vi "main.vi"(0 "Test Pins":T9, 1 "Caller Information":T6, 5 "Test Inputs":T10={"Input Voltage Vin1 in V"=0.0, "Input Voltage Vin2 in V"=0.0, "Duration of the pulse in s"=0.5, "Nominal Output Voltage in V"=0.0, "Ref Voltage level for Settling Time Calc"=0.1, "% of Vnom for Settling Time Calc"=10.0, "Settling Time Calc Option"=enum."Voltage Level ", "Advance Setting"={"Prepare"={"Load SMU Output Function"=enum."VoltageSource"}}, "Save Transient Graph?"=TRUE, "Load Current in A"=0.0, "Save Scope Raw Data?"=FALSE, "Delay - t1 (s)"=0.25, "Delay - t2 (s)"=0.25, "Auto Scale Y-Axis?"=TRUE}, 11 "error in":errorcluster) -> (4 "Test Results":T15 {"Second Edge - Settling Time in s" format="%#.5p"; "First Edge - Settling Time in s" format="%#.5p"; "Actual Sample Rate" format="%#.5g"}, 15 "error out":errorcluster)   [LabVIEW 2020, in "LDO Line Transient.lvlib"]
doc: "<b>Caller</b> Information is input for framework components. Mode should be set to <b>Automation</b> when running from TestStand. Sequence Context should be set to <b>ThisContext</b> when running from TestStand. The values will be updated everytime the setting is applied using \"Edit\" dialog.\n\n<b>Test Pins</b> is names of pins available in the pinmap file. Provide the right pins for the required functionality.\n\n<b>Test Inputs</b> is input required for the measurement to perform.\n\n<b>error in</b> is meant for the sequencing. <b>error in</b> should be <b>no error</b> always.\n\n<b>Test Results</b> contains all the measured data during the measurement and processed results.\n\n<b>error out</b> contains the error occured during measurement.\n\nCheck measurement documentation for more information (<Program Files>\\Soliton Technologies\\MeasurementSuite\\CodeModules\\LDO\\LDO Line Transient.pdf)"
uses:
  LDO Line Transient.lvlib
  Typedefs/Test Results.ctl
  Typedefs/Test Inputs.ctl
  Typedefs/Settling Time Calc Option.ctl
  Typedefs/Advance Settings.ctl
  Typedefs/Adv Settings Setup Instr.ctl
  Reusables/Instrument APIs/Load Output Function.ctl
  <userlib>/_Soliton/Measurement Suite/Reusables/Plugin Common/Typedefs/Caller Events.ctl
  <userlib>/_Soliton/Measurement Suite/Reusables/Plugin Common/Typedefs/Caller Information.ctl
  <userlib>/_Soliton/Measurement Suite/Reusables/Plugin Common/Typedefs/Caller Mode.ctl
  Typedefs/Test Pins.ctl
  Typedefs/Pin Dropdown.ctl
  <userlib>/_Soliton/Measurement Suite/Reusables/Plugin Common/Typedefs/Termination Monitor Info.ctl
  Typedefs/Test Results - Output Voltage Params.ctl
  Typedefs/Test Results - Input Voltage Params.ctl
  Reusables/UI/Progress Monitor/Progress Monitor Option.ctl
  <vilib>/Utility/miscctls.llb/LVMajorAndMinorColorsTypeDef.ctl
  <instrlib>/niDCPower/nidcpower.llb/niDCPower Wait For Event - Event.ctl
  <instrlib>/niDCPower/nidcpower.llb/niDCPower Source Mode.ctl
  <instrlib>/niDCPower/nidcpower.llb/niDCPower Output Function.ctl
  <instrlib>/niScope/Controls/niScope scalar measurement.ctl
  <vilib>/Utility/error.llb/DialogType.ctl
  98935dad-41b4-4920-b943-01b05448cf2f.vi
  d648f1df-a8d9-4085-9eb0-24252e83c66e.vi
  c145c5dd-ae3b-4a85-a29b-a78c16d0dffa.vi
  92dab295-f5c3-455d-a51b-398903a4b680.vi
  64e7d395-4f1e-47d2-aa56-89bf032ac911.vi
  a2cb5138-c738-477a-b5c4-3cdfd9a525fc.vi
  e1ff1980-5b52-43e3-809b-8f211f405b25.vi
  49732470-67c5-4264-8b59-91d7a6bf13ef.vi
  7d547965-4422-4a29-bcba-22e7343550fa.vi
  f054ac9e-285a-43ff-a938-075fc082fc86.vi
  bb3e62c4-a2c2-4505-9438-f842dd651d6c.vi
  ce2ee1e5-697c-4608-b941-8c9b0f21ffd9.vi
  217e438d-a1ad-49ce-9dcd-d015b5ab8206.vi
  20f14550-4756-4008-9ed5-c13eed5fd878.vi
  <userlib>/_Soliton/Measurement Suite/Reusables/InstrumentSessionAPIs/SessionManagerApiPath.vi
  <vilib>/Utility/sysdir.llb/Get System Directory.vi
  <vilib>/Utility/LVLibp/Get Exported File Path.vi
  <userlib>/_Soliton/Measurement Suite/Reusables/Errors/Error 6001.vi
  <instrlib>/niScope/Acquire/Fetch/niScope Multi Fetch Cluster.vi
  <instrlib>/niScope/Measurements/niScope Fetch Measurement.vi
  <userlib>/_Soliton/Measurement Suite/Reusables/Plugin Common/Plugin Common.lvlib
  <userlib>/_Soliton/Measurement Suite/Reusables/Queue Driver/Plugin Queue Driver.lvlib
panel:
  out "Progress":i32(slide) scale=-1.0..0.1
  in  "Terminate":bool
  in  "Run":bool caption="Measure"
  in  "Exit":bool
  out "Header":string
  in  "Tab Enum":T1(radio)
  out "Tab Control":T2(tab)
  in  "SystemSetup":T4={"Set Input Voltage"={"PinStatus"=0, "PinName"="", "Info"=TRUE}, "Measure Input Voltage"={"PinStatus"=0, "PinName"="", "Info"=TRUE}, "Measure Output Voltage"={"PinStatus"=0, "PinName"="", "Info"=TRUE}, "Set Load Current"={"PinStatus"=0, "PinName"="", "Info"=TRUE}}
  out "Sequence Timeout":dbl caption="Sequence Timeout (s)" format="%#.5p"
  in  "Scope Reference Position":dbl format="%#_1f"
  in  "Delay - t2 (s)":dbl=0.25 format="%#_6p"
  in  "Delay - t1 (s)":dbl=0.25 format="%#_6p"
  in  "Load Current (A)":dbl format="%#_6p"
  in  "Voltage to settle above Vnom (V)":dbl=0.1 format="%#_6p"
  in  "Percentage of Vnom (%)":dbl=10.0 caption="Percentage of nominal voltage (%)" format="%#_6f"
  in  "Input Voltage 1 - Vin1 (V)":dbl format="%#_6p"
  in  "Settling Time Calculation":enum32{"Item 0", "Item 1"}(radio)
  in  "Duration of the pulse (s)":dbl=0.5 format="%#_6p"
  in  "Input Voltage 2 - Vin2 (V)":dbl format="%#_6p"
  in  "Nominal Output Voltage (V)":dbl format="%#_6p"
  in  "Advanced Settings":bool
  in  "Auto Scale Y-Axis?":bool=TRUE
  in  "Save Scope Raw Data?":bool=TRUE
  out "Second Edge - Peak Voltage (V)":dbl caption="Peak Voltage (V)" format="%#.6p"
  out "Second Edge - Settling Time (s)":dbl format="%#.5p"
  out "First Edge - Peak Voltage (V)":dbl caption="Peak Voltage (V)" format="%#.6p"
  out "Line Transient":T5(graph)
  in  "Take Transient snapshot?":bool=TRUE
  out "Transient Input Voltage":waveform(dbl)(graph)
  out "Line Transient":T5(graph)
  out "First Edge - Settling Time (s)":dbl format="%#.5p"
  in  "ErrorOccured":errorcluster
  in  "Caller Events":T8
  in  "DataLogPath":path
  # "Supports NIScopeInstrument"
  # "Supports NIScopeInstrument"
  # "Supports NIDCPowerInstrument"
  # "Supports NIDCPowerInstrument"
  # "Settling Time Calculation"
  # "Settling Time is defined as the time taken for the output voltage to recover\nto the LDO nominal output voltage."
  # "Time taken for output voltage to settle to (Choose one below)"
  # "Line Transient"
  # "Output Voltage"
  # "Load SMU"
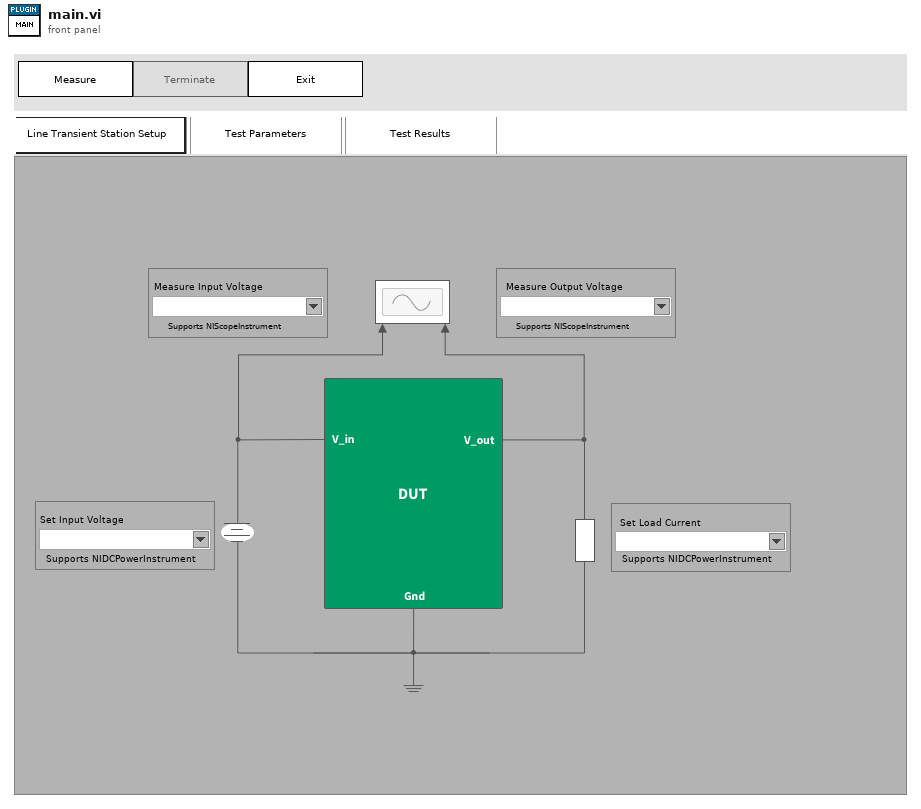
[diagram p1: front panel]
types:
  T1 = enum32{"Station Setup", "Test Parameters", "Test Results"}
  T2 = enum32{"Station Setup", "Test Parameters", "Test Results", "Debug"}
  T3 = typedef "LDO Line Transient.lvlib/Pin Dropdown.ctl" = cluster{"PinStatus":u16, "PinName":string, "Info":bool}
  T4 = cluster{"Set Input Voltage":T3, "Measure Input Voltage":T3, "Measure Output Voltage":T3, "Set Load Current":T3}
  T5 = cluster{"relativeInitialX":dbl, "xIncrement":dbl, "wfm":dbl[]}[]
  T6 = typedef "Plugin Common.lvlib/Caller Information.ctl" = cluster{"Mode":T7, "Sequence Context":refnum<k7>}
  T7 = typedef "Plugin Common.lvlib/Caller Mode.ctl" = enum16{"Standalone", "Automation", "MeasurementSuite"}
  T8 = typedef "Plugin Common.lvlib/Caller Events.ctl" = cluster{"Caller Event":refnum<user-event>}
  T9 = typedef "LDO Line Transient.lvlib/Test Pins.ctl" = cluster{"Set Input Voltage":string, "Set Load Current":string, "Measure Input Voltage":string, "Measure Output Voltage":string}
  T10 = typedef "LDO Line Transient.lvlib/Test Inputs.ctl" = cluster{"Input Voltage Vin1 in V":dbl, "Input Voltage Vin2 in V":dbl, "Duration of the pulse in s":dbl, "Nominal Output Voltage in V":dbl, "Ref Voltage level for Settling Time Calc":dbl, "% of Vnom for Settling Time Calc":dbl, "Settling Time Calc Option":T11, "Advance Setting":T12, "Save Transient Graph?":bool, "Load Current in A":dbl, "Save Scope Raw Data?":bool, "Delay - t1 (s)":dbl, "Delay - t2 (s)":dbl, "Auto Scale Y-Axis?":bool}
  T11 = typedef "LDO Line Transient.lvlib/Settling Time Calc Option.ctl" = enum16{"Voltage Level ", "Percentage of Vnom"}
  T12 = typedef "LDO Line Transient.lvlib/Advance Settings.ctl" = cluster{"Prepare":T13}
  T13 = typedef "LDO Line Transient.lvlib/Adv Settings Setup Instr.ctl" = cluster{"Load SMU Output Function":T14}
  T14 = typedef "Load Output Function.ctl" = enum16{"VoltageSource", "CurrentSource"}
  T15 = typedef "LDO Line Transient.lvlib/Test Results.ctl" = cluster{"Output Voltage Measured":cluster{"relativeInitialX":dbl, "xIncrement":dbl, "wfm":dbl[]}, "Input Voltage Measured":cluster{"relativeInitialX":dbl, "xIncrement":dbl, "wfm":dbl[]}, "Actual Sample Rate":dbl, "First Edge - Settling Time in s":dbl, "Second Edge - Settling Time in s":dbl}
  T16 = typedef "Plugin Common.lvlib/Termination Monitor Info.ctl" = cluster{"Caller Information":T6, "Execution":refnum<k7>, "Termination Monitor":refnum<k7>, "Type":string, "Plugin Name":string}
  T17 = typedef "LDO Line Transient.lvlib/Test Results - Output Voltage Params.ctl" = cluster{"First Edge - Settling Time (s)":dbl, "First Edge - Peak Voltage (V)":dbl, "Second Edge - Settling Time (s)":dbl, "Second Edge - Peak Voltage (V)":dbl, "Vmax":dbl, "Vmin":dbl}
  T18 = typedef "LDO Line Transient.lvlib/Test Results - Input Voltage Params.ctl" = cluster{"Vmax":dbl, "Vmin":dbl}
  T19 = cluster{"Termination Monitor Info":T16, "Test Inputs":T10, "Test Results":T15, "Test Results[][]":string[][], "Test Pins":T9, "Logger Folder Path":path, "Valid Logger Path?":bool, "Logger File Path":path, "Waveform for settling time analysis":dbl[], "Min delay for Reference Position":u32, "Output Voltage Coupling":i32, "Input Voltage Waveform":dbl[], "Input Voltage Source Delay":dbl[], "Output Voltage Params":T17, "Input Voltage Params":T18, "UI Ctls":refnum<vi>[]}
  T20 = typedef "Progress Monitor Option.ctl" = enum16{"State Array Init", "Get State Index"}
  T21 = enum8{"Enabled", "Disabled", "Disabled and Grayed Out"}
  T22 = cluster{"Set Iload":T3, "Set Vin":T3, "Capture Vout":T3, "Capture Vin":T3}
  T23 = typedef "LVMajorAndMinorColorsTypeDef.ctl" = cluster{"Major Color":u32, "Minor Color":u32}
  T24 = cluster{"relativeInitialX":dbl, "xIncrement":dbl, "wfm":dbl[]}
  T25 = typedef "niDCPower Wait For Event - Event.ctl" = i32
  T26 = typedef "niDCPower Output Function.ctl" = i32
  T27 = typedef "niDCPower Source Mode.ctl" = i32
  T28 = typedef "niScope scalar measurement.ctl" = i32
  T29 = typedef "DialogType.ctl" = u16
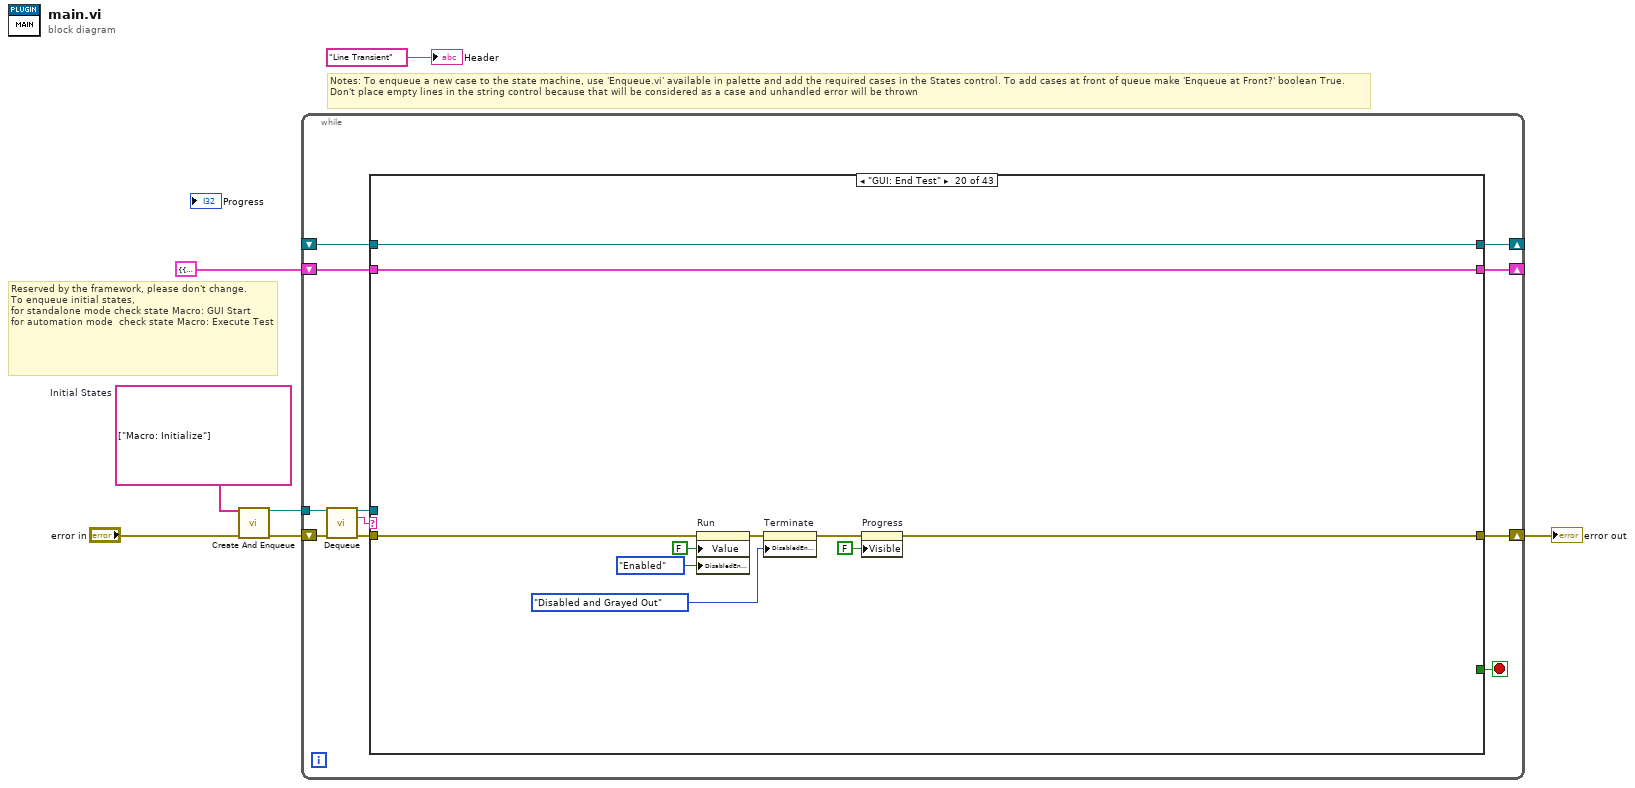
[diagram p0: block diagram]
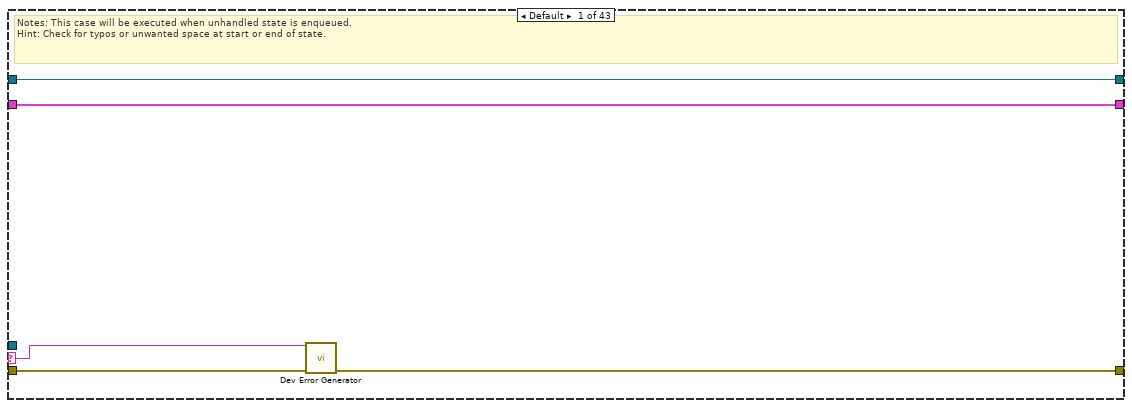
[diagram p2: hidden frame]
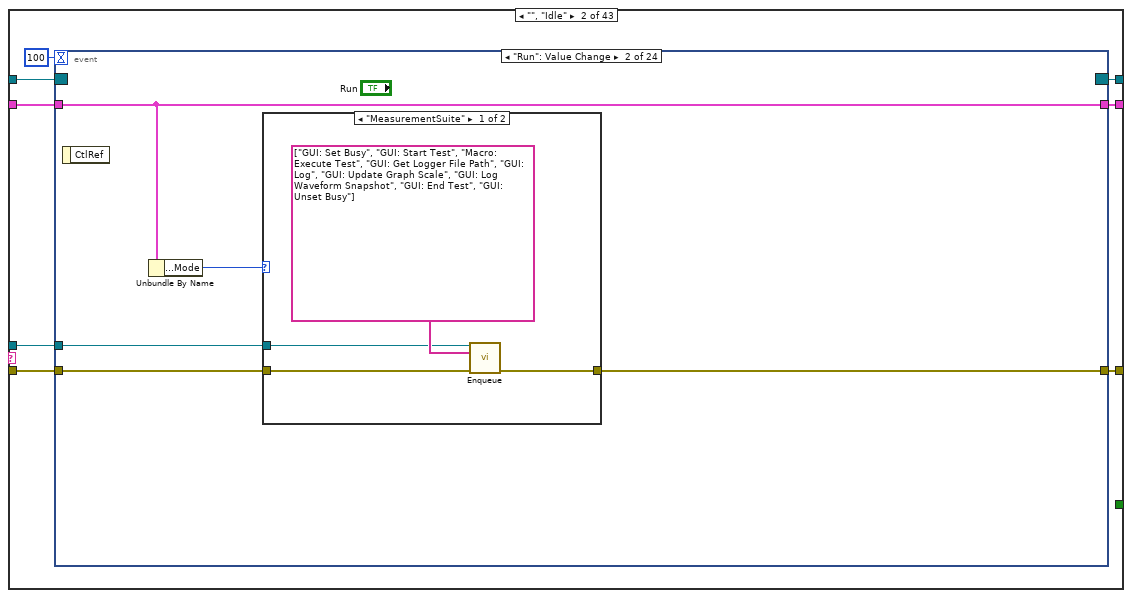
[diagram p3: hidden frame]
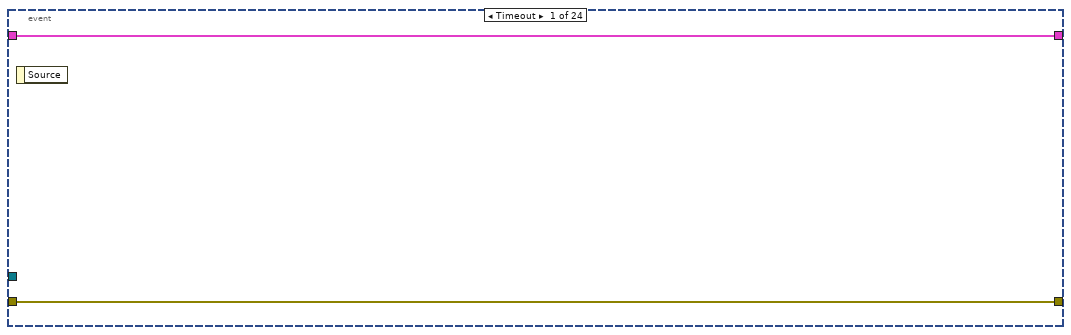
[diagram p4: hidden frame]
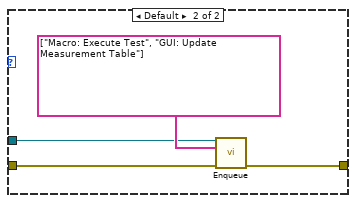
[diagram p5: hidden frame]
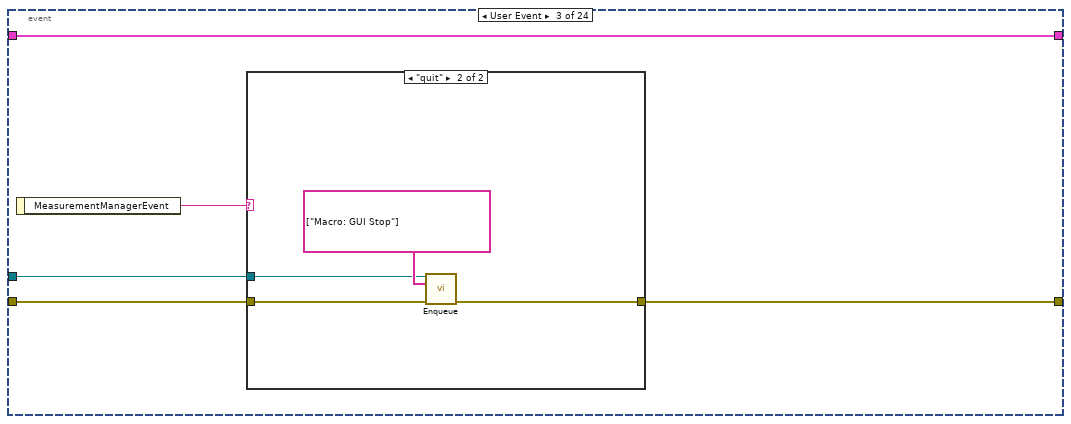
[diagram p6: hidden frame]
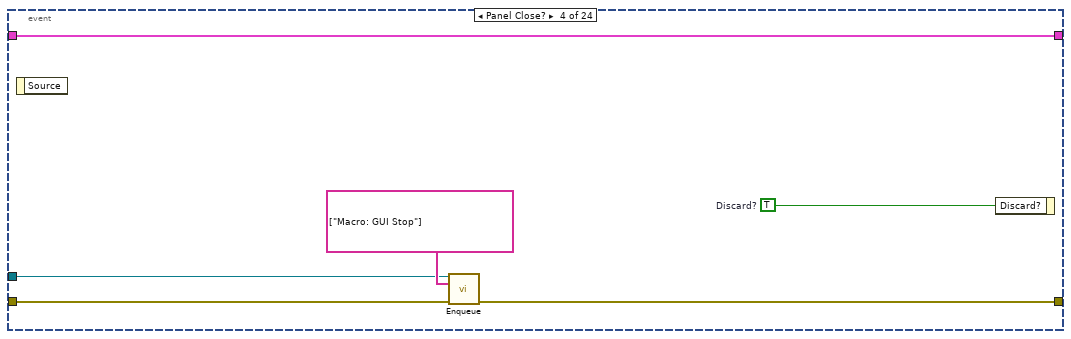
[diagram p8: hidden frame]
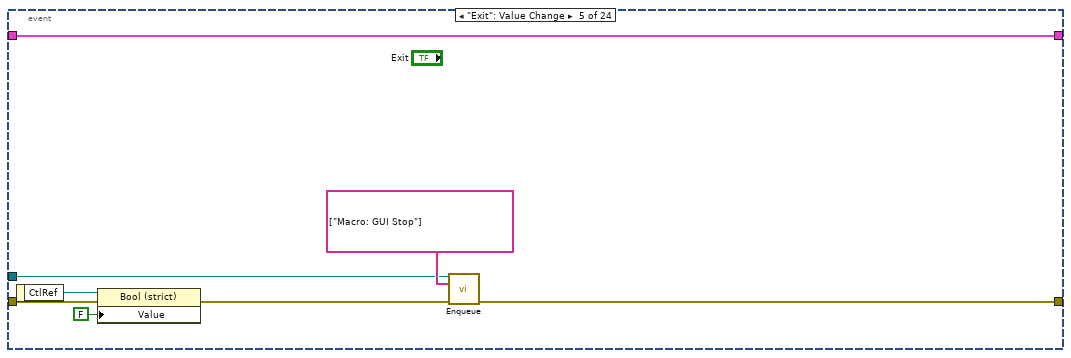
[diagram p9: hidden frame]
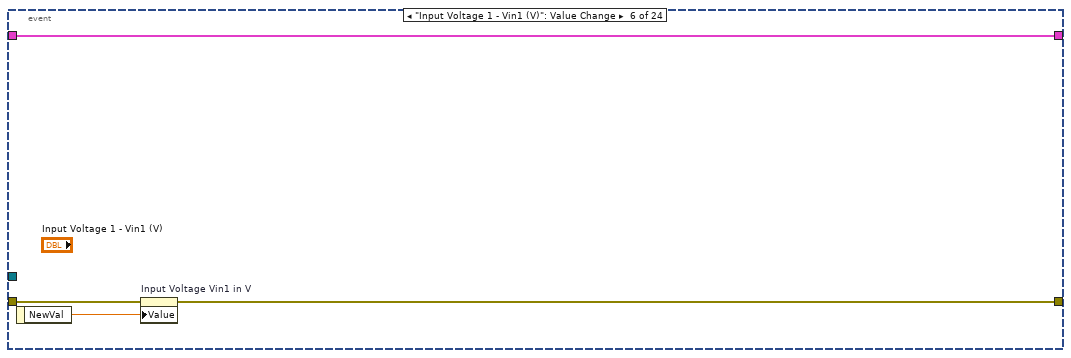
[diagram p10: hidden frame]
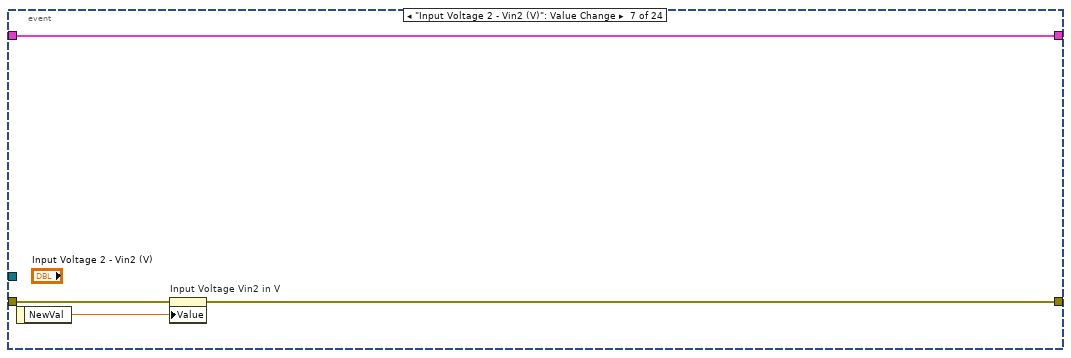
[diagram p11: hidden frame]
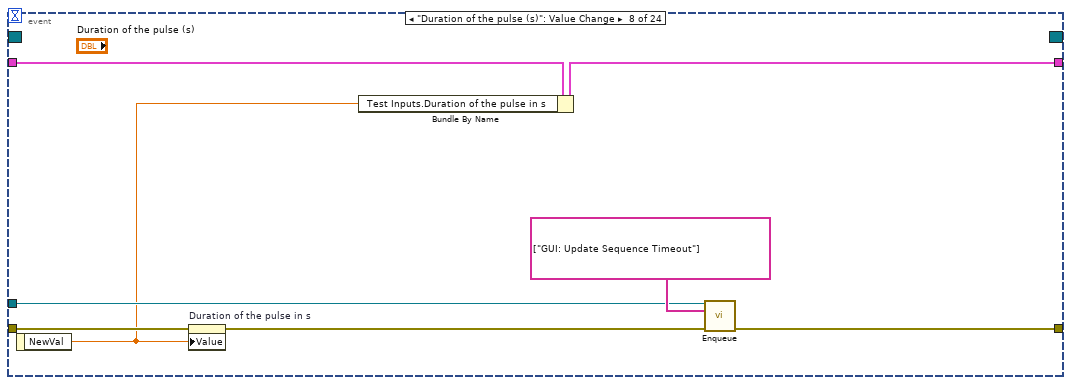
[diagram p12: hidden frame]
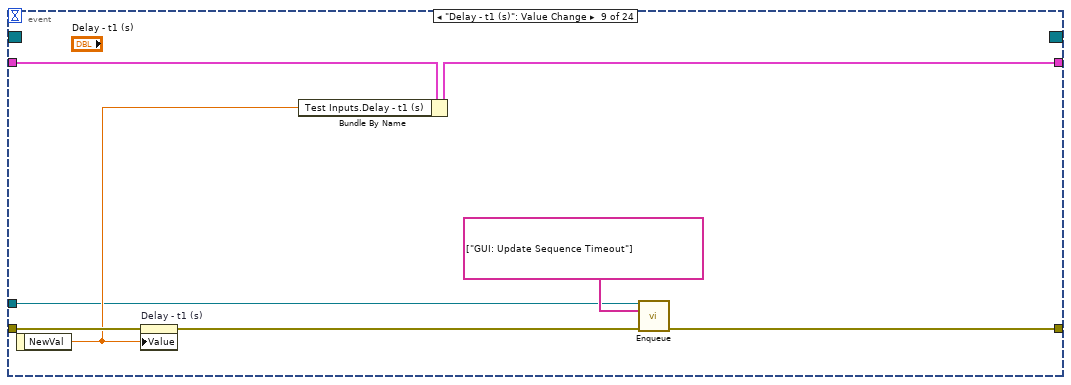
[diagram p13: hidden frame]
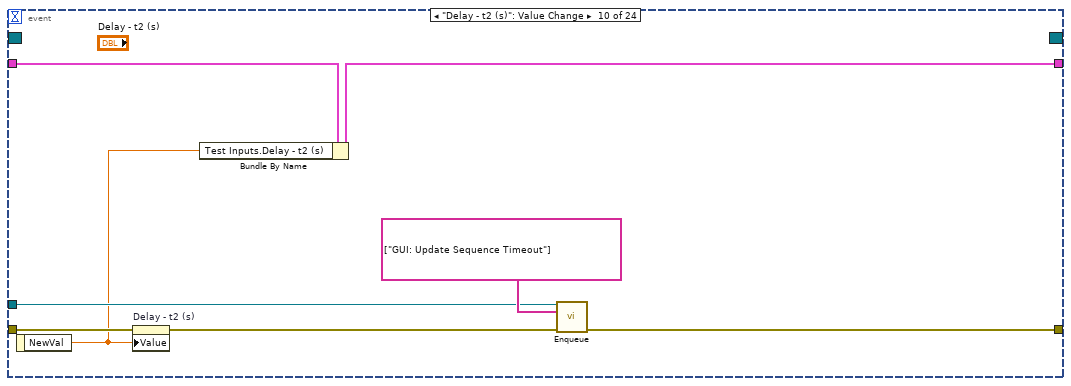
[diagram p14: hidden frame]
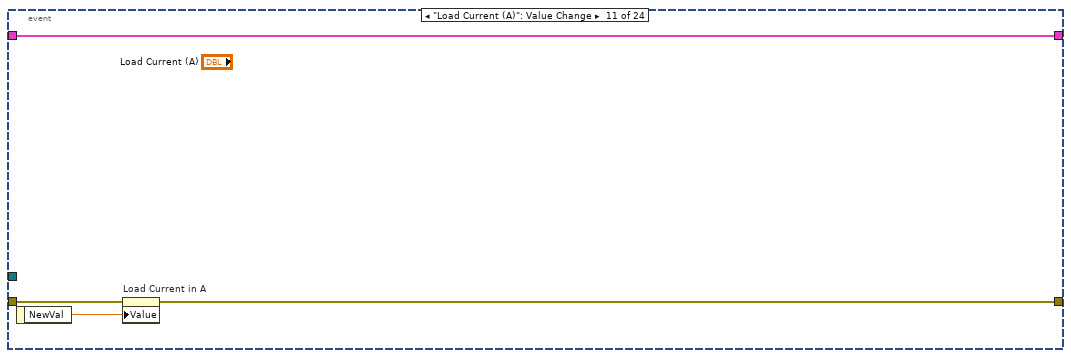
[diagram p15: hidden frame]
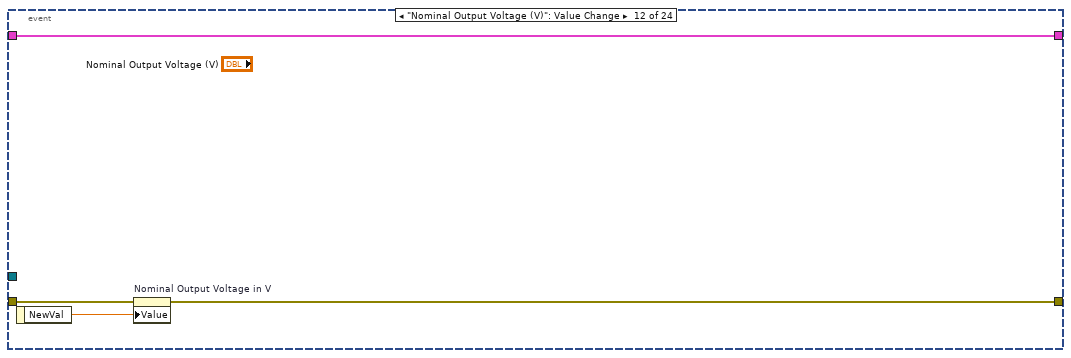
[diagram p16: hidden frame]
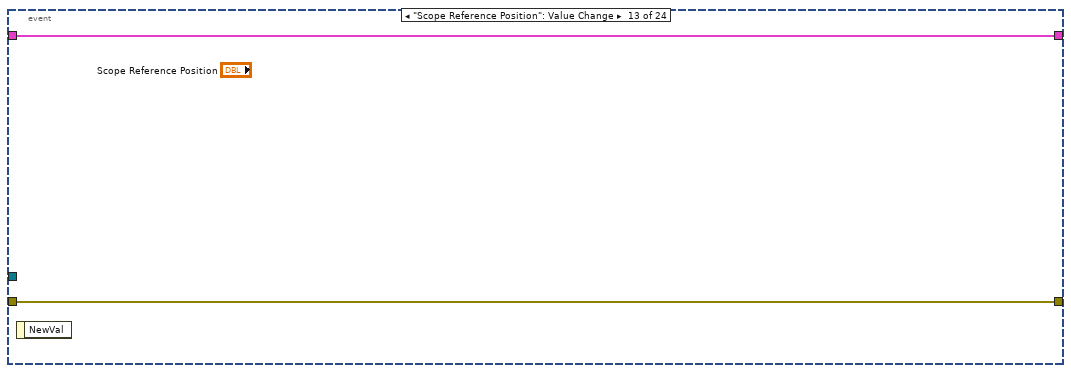
[diagram p17: hidden frame]
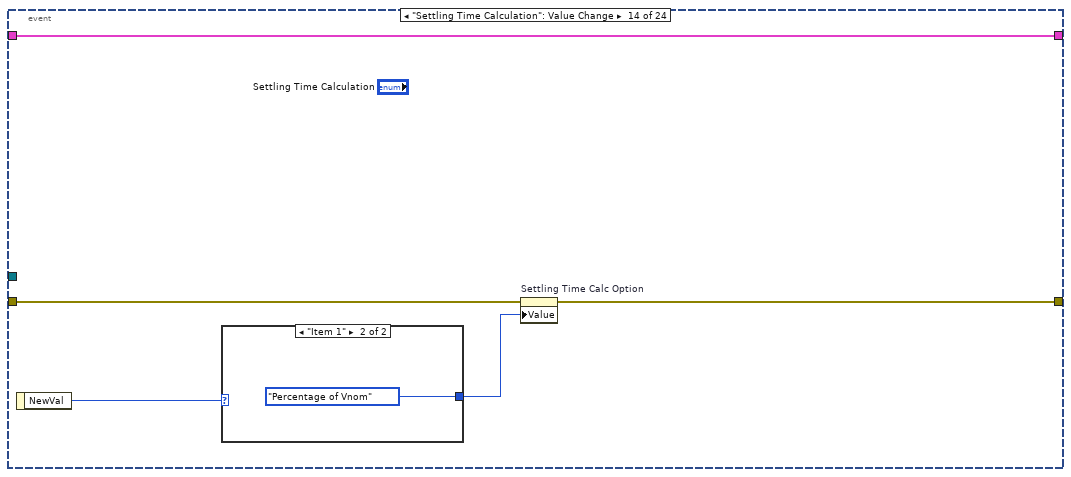
[diagram p18: hidden frame]
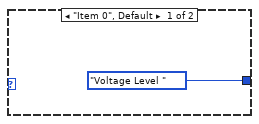
[diagram p19: hidden frame]
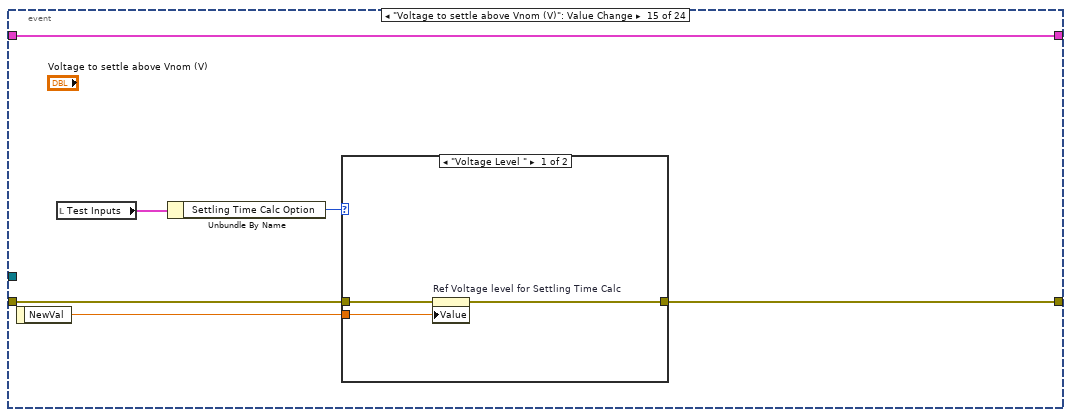
[diagram p20: hidden frame]
diagram:
  w7 = string[] ["Macro: Initialize"]  # Initial States
  # "Notes: To enqueue a new case to the state machine, use 'Enqueue.vi' available in palette and add the required cases in the States control. To add cases at front of queue make 'Enqueue at Front?' boolean True. Don't place empty lines in the string control because that will be considered as a case and unhandled error will be thrown"
  # "Reserved by the framework, please don't change. \nTo enqueue initial states,\nfor standalone mode check state Macro: GUI Start\nfor automation mode  check state Macro: Execute Test"
  n1 = call <userlib>:"Create And Enqueue.vi"("Initial States"=w7, "error in (no error)"="error in") -> ("Queue out"=w5:refnum<queue>, "error out"=w3:errorcluster)  [unwired: 12 in]
  n2 = while {
    shift-right: [w18] -> w4
    shift-left: w3 -> [w16]
    shift-right: [w14] -> _
    shift-left: T19 {"Termination Monitor Info"={"Caller Information"={"Mode"=enum."Standalone", "Sequence Context"=refnum}, "Execution"=refnum, "Termination Monitor"=refnum, "Type"="", "Plugin Name"=""}, "Test Inputs"={"Input Voltage Vin1 in V"=0.0, "Input Voltage Vin2 in V"=0.0, "Duration of the pulse in s"=0.0, "Nominal Output Voltage in V"=0.0, "Ref Voltage level for Settling Time Calc"=0.0, "% of Vnom for Settling Time Calc"=0.0, "Settling Time Calc Option"=enum."Voltage Level ", "Advance Setting"={"Prepare"={"Load SMU Output Function"=enum."VoltageSource"}}, "Save Transient Graph?"=FALSE, "Load Current in A"=0.0, "Save Scope Raw Data?"=FALSE, "Delay - t1 (s)"=0.0, "Delay - t2 (s)"=0.0, "Auto Scale Y-Axis?"=FALSE}, "Test Results"={"Output Voltage Measured"={"relativeInitialX"=0.0, "xIncrement"=0.0, "wfm"=[]}, "Input Voltage Measured"={"relativeInitialX"=0.0, "xIncrement"=0.0, "wfm"=[]}, "Actual Sample Rate"=0.0, "First Edge - Settling Time in s"=0.0, "Second Edge - Settling Time in s"=0.0}, "Test Results[][]"=[], "Test Pins"={"Set Input Voltage"="", "Set Load Current"="", "Measure Input Voltage"="", "Measure Output Voltage"=""}, "Logger Folder Path"=path "", "Valid Logger Path?"=FALSE, "Logger File Path"=path "", "Waveform for settling time analysis"=[], "Min delay for Reference Position"=0, "Output Voltage Coupling"=0, "Input Voltage Waveform"=[], "Input Voltage Source Delay"=[], "Output Voltage Params"={"First Edge - Settling Time (s)"=0.0, "First Edge - Peak Voltage (V)"=0.0, "Second Edge - Settling Time (s)"=0.0, "Second Edge - Peak Voltage (V)"=0.0, "Vmax"=0.0, "Vmin"=0.0}, "Input Voltage Params"={"Vmax"=0.0, "Vmin"=0.0}, "UI Ctls"=[]} -> [w13]
    tunnel: w5 -> [w12]
    shift-right: [w9] -> _
    shift-left: _ -> [w10]
    stop <- w17 stop-if-true
    n3 = call <userlib>:"Dequeue.vi"("Queue in"=w12, "error in (no error)"=w16) -> ("Queue out"=w11:refnum<queue>, "Dequeued State"=w8:string, "error out"=w15:errorcluster)  [unwired: 11 in]
    n4 = case shown="\"GUI: End Test\"" w8 {
      selector: w8 -> [w21 _ _ _ _ _ _ _ _ _ _ _ _ _ _ _ w423 w439 _ _ _ _ _ _ _ w508 w529 w541 w574 w588 w598 w615 w673 w701 w732 w756 w777 w806 w825 w830 _ _ _]
      tunnel: w15 -> [w20 w28 w227 w236 w251 w257 w264 w269 w312 w323 w327 w330 w334 w363 w378 w389 w424 w440 w456 w467 w476 w487 w492 w499 w504 w506 w530 w542 w575 w589 w599 w616 w674 w702 w733 w757 w778 w807 w826 w831 w838 w845 w863]
      tunnel: [w22 w29 w227 w239 w247 w258 w265 w269 w292 w321 w325 w330 w333 w364 w376 w390 w428 w444 w457 w468 w475 w487 w493 w500 w504 w509 w533 w540 w563 w590 w607 w634 w689 w721 w734 w758 w772 w795 w824 w832 w838 w843 w857] -> w18
      tunnel: [_ _ _ _ _ _ _ _ _ _ _ _ _ _ _ _ _ _ _ _ _ _ _ _ _ _ _ _ _ _ _ _ _ _ _ _ _ _ _ _ _ w840 TRUE] -> w17
      tunnel: [w23 w31 w226 w229 w252 w259 w266 w268 w289 w322 w326 w329 w332 w365 w382 w388 w427 w443 w464 w474 w477 w486 w491 w498 w503 w512 w535 w545 w556 w593 w606 w624 w687 w718 w737 w761 w792 w811 w828 w835 w837 w842 w864] -> w14
      tunnel: w13 -> [w23 w30 w226 w240 w252 w259 w266 w268 w317 w322 w326 w329 w331 w365 w382 w388 w427 w443 w464 w474 w477 w486 w490 w497 w503 w519 w535 w545 w555 w592 w606 w623 w686 w717 w736 w760 w792 w811 w828 w835 w837 w842 w864]
      tunnel: w11 -> [_ w24 _ w238 w250 w255 w262 _ _ _ _ _ _ _ _ _ _ _ _ _ _ _ _ _ _ _ _ _ _ _ _ _ _ _ _ _ _ _ _ _ _ w839 w862]
      tunnel: w10 -> [w19 w26 w225 w237 w249 w254 w261 w267 w316 _ w324 w328 w339 w366 w383 w395 w434 w450 w463 w473 w484 w485 w494 w501 w502 w517 w536 w546 w583 w597 w614 w638 w698 w731 w743 w762 w793 w817 w829 w834 w836 w844 w861]
      tunnel: [w19 w25 w225 w237 w249 w254 w261 w267 w316 w320 w324 w328 w339 w366 w383 w395 w434 w450 w463 w473 w484 w485 w494 w501 w502 w517 w536 w546 w583 w597 w614 w638 w698 w731 w743 w762 w793 w817 w829 w834 w836 w844 w861] -> w9
      frame Default {
        # "Notes: This case will be executed when unhandled state is enqueued. \nHint: Check for typos or unwanted space at start or end of state."
        n5 = call <userlib>:"Dev Error Generator.vi"("State"=w21, "error in (no error)"=w20) -> ("error out"=w22:errorcluster)  [unwired: 13 in]
      }
      frame "", "Idle" {
        n6 = event shown="[1] \"Run\": Value Change" {
          selector: w26 -> [_ _ _ _ _ _ _ _ _ _ _ _ _ _ _ _ _ _ _ _ _ _ _ _]
          dyn-events: [_ _ _ _ _ _ _ _ _ _ _ _ _ _ _ _ _ _ _ _ _ _ _ _] -> w25
          timeout: 100 -> [_ _ _ _ _ _ _ _ _ _ _ _ _ _ _ _ _ _ _ _ _ _ _ _]
          tunnel: [w33 w35 w51 w62 w70 w74 w78 w81 w93 w96 w106 w110 w112 w117 w125 w136 w147 w151 w155 w158 w174 w212 w217 w222] -> w31
          tunnel: w30 -> [w33 w35 w51 w62 w70 w74 w78 w80 w92 w95 w106 w110 w112 w117 w125 w136 w147 w151 w155 w162 w173 w211 w217 w221]
          tunnel: [w32 w38 w49 w59 w68 w73 w77 w83 w88 w99 w104 w109 w111 w114 w123 w133 w145 w149 w153 w160 w176 w191 w216 w219] -> w29
          tunnel: w28 -> [w32 w37 w50 w58 w67 w72 w76 w86 w94 w102 w105 w108 w111 w115 w124 w132 w146 w150 w154 w159 w177 w187 w216 w224]
          tunnel: w24 -> [_ w36 w47 w57 w66 _ _ w82 w87 w98 _ _ _ _ _ _ _ _ _ _ _ _ _ _]
          event Timeout {
            n7 = event-data() -> ()  [unwired: 1 in, 1 out]
          }
          event "Run": Value Change {
            n8 = event-data() -> ()  [unwired: 1 in, 1 out]
            n9 = Unbundle By Name(w35) -> ("Termination Monitor Info.Caller Information.Mode"=w34:T7)
            n10 = case shown="\"MeasurementSuite\"" w34 {
              tunnel: [w41 w45] -> w38
              tunnel: w37 -> [w40 w44]
              tunnel: w36 -> [w39 w43]
              frame "MeasurementSuite" {
                n11 = call <userlib>:"Enqueue.vi"("Queue in"=w39, "States"=string[] ["GUI: Set Busy", "GUI: Start Test", "Macro: Execute Test", "GUI: Get Logger File Path", "GUI: Log", "GUI: Update Graph Scale", "GUI: Log Waveform Snapshot", "GUI: End Test", "GUI: Unset Busy"], "error in (no error)"=w40) -> ("error out"=w41:errorcluster)  [unwired: 11 in, 1 out]
              }
              frame Default {
                n12 = call <userlib>:"Enqueue.vi"("Queue in"=w43, "States"=string[] ["Macro: Execute Test", "GUI: Update Measurement Table"], "error in (no error)"=w44) -> ("error out"=w45:errorcluster)  [unwired: 11 in, 1 out]
              }
            }
          }
          event User Event {
            n13 = event-data() -> ("MeasurementManagerEvent"=w48:string)  [unwired: 1 in]
            n14 = case shown="\"quit\"" w48 {
              tunnel: [w52 w53] -> w49
              tunnel: w50 -> [w52 w55]
              tunnel: w47 -> [_ w54]
              frame Default {
              }
              frame "quit" {
                n15 = call <userlib>:"Enqueue.vi"("Queue in"=w54, "States"=string[] ["Macro: GUI Stop"], "error in (no error)"=w55) -> ("error out"=w53:errorcluster)  [unwired: 11 in, 1 out]
              }
            }
          }
          event Panel Close? {
            w61 = TRUE  # Discard?
            n16 = event-data() -> ()  [unwired: 1 in, 1 out]
            n17 = call <userlib>:"Enqueue.vi"("Queue in"=w57, "States"=string[] ["Macro: GUI Stop"], "error in (no error)"=w58) -> ("error out"=w59:errorcluster)  [unwired: 11 in, 1 out]
            n18 = event-data("Discard?"=w61) -> ()  [unwired: 1 in, 1 out]
          }
          event "Exit": Value Change {
            n19 = event-data() -> ("CtlRef"=w64:refnum<vi>)  [unwired: 1 in]
            n20 = property class="Bool (strict)"(reference=w64, error in=w67, "Value"=FALSE) -> (error out=w65:errorcluster)  [unwired: 1 out]
            n21 = call <userlib>:"Enqueue.vi"("Queue in"=w66, "States"=string[] ["Macro: GUI Stop"], "error in (no error)"=w65) -> ("error out"=w68:errorcluster)  [unwired: 11 in, 1 out]
          }
          event "Input Voltage 1 - Vin1 (V)": Value Change {
            n22 = event-data() -> ("NewVal"=w71:dbl)  [unwired: 1 in]
            n23 = property on="Input Voltage Vin1 in V" class="DigNum (strict)"(error in=w72, "Value"=w71) -> (error out=w73:errorcluster)  [unwired: 1 in, 1 out]
          }
          event "Input Voltage 2 - Vin2 (V)": Value Change {
            n24 = event-data() -> ("NewVal"=w75:dbl)  [unwired: 1 in]
            n25 = property on="Input Voltage Vin2 in V" class="DigNum (strict)"(error in=w76, "Value"=w75) -> (error out=w77:errorcluster)  [unwired: 1 in, 1 out]
          }
          event "Duration of the pulse (s)": Value Change {
            n26 = event-data() -> ("NewVal"=w79:dbl)  [unwired: 1 in]
            n27 = property on="Duration of the pulse in s" class="DigNum (strict)"(error in=w86, "Value"=w79) -> (error out=w84:errorcluster)  [unwired: 1 in, 1 out]
            n28 = Bundle By Name(cluster=w80, "Test Inputs.Duration of the pulse in s"=w79) -> (w81:T19)
            n29 = call <userlib>:"Enqueue.vi"("Queue in"=w82, "States"=string[] ["GUI: Update Sequence Timeout"], "error in (no error)"=w84) -> ("error out"=w83:errorcluster)  [unwired: 11 in, 1 out]
          }
          event "Delay - t1 (s)": Value Change {
            n30 = event-data() -> ("NewVal"=w91:dbl)  [unwired: 1 in]
            n31 = property on="Delay - t1 (s)" class="DigNum (strict)"(error in=w94, "Value"=w91) -> (error out=w89:errorcluster)  [unwired: 1 in, 1 out]
            n32 = Bundle By Name(cluster=w92, "Test Inputs.Delay - t1 (s)"=w91) -> (w93:T19)
            n33 = call <userlib>:"Enqueue.vi"("Queue in"=w87, "States"=string[] ["GUI: Update Sequence Timeout"], "error in (no error)"=w89) -> ("error out"=w88:errorcluster)  [unwired: 11 in, 1 out]
          }
          event "Delay - t2 (s)": Value Change {
            n34 = event-data() -> ("NewVal"=w97:dbl)  [unwired: 1 in]
            n35 = property on="Delay - t2 (s)" class="DigNum (strict)"(error in=w102, "Value"=w97) -> (error out=w100:errorcluster)  [unwired: 1 in, 1 out]
            n36 = Bundle By Name(cluster=w95, "Test Inputs.Delay - t2 (s)"=w97) -> (w96:T19)
            n37 = call <userlib>:"Enqueue.vi"("Queue in"=w98, "States"=string[] ["GUI: Update Sequence Timeout"], "error in (no error)"=w100) -> ("error out"=w99:errorcluster)  [unwired: 11 in, 1 out]
          }
          event "Load Current (A)": Value Change {
            n38 = event-data() -> ("NewVal"=w103:dbl)  [unwired: 1 in]
            n39 = property on="Load Current in A" class="DigNum (strict)"(error in=w105, "Value"=w103) -> (error out=w104:errorcluster)  [unwired: 1 in, 1 out]
          }
          event "Nominal Output Voltage (V)": Value Change {
            n40 = event-data() -> ("NewVal"=w107:dbl)  [unwired: 1 in]
            n41 = property on="Nominal Output Voltage in V" class="DigNum (strict)"(error in=w108, "Value"=w107) -> (error out=w109:errorcluster)  [unwired: 1 in, 1 out]
          }
          event "Scope Reference Position": Value Change {
            n42 = event-data() -> ()  [unwired: 1 in, 1 out]
          }
          event "Settling Time Calculation": Value Change {
            n43 = event-data() -> ("NewVal"=w116:enum32{"Item 0", "Item 1"})  [unwired: 1 in]
            n44 = case shown="\"Item 1\"" w116 {
              tunnel: [Settling_Time_Calc_Option."Voltage Level " ("Value") Settling_Time_Calc_Option."Percentage of Vnom" ("Value")] -> w113
              frame "Item 0", Default {
              }
              frame "Item 1" {
              }
            }
            n45 = property on="Settling Time Calc Option" class="Enum (strict)"(error in=w115, "Value"=w113) -> (error out=w114:errorcluster)  [unwired: 1 in, 1 out]
          }
          event "Voltage to settle above Vnom (V)": Value Change {
            n46 = event-data() -> ("NewVal"=w120:dbl)  [unwired: 1 in]
            n47 = local read "Test Inputs"() -> (w122:T10)
            n48 = Unbundle By Name(w122) -> ("Settling Time Calc Option"=w121:T11)
            n49 = case shown="\"Voltage Level \"" w121 {
              tunnel: w124 -> [w128 w129]
              tunnel: [w127 w129] -> w123
              tunnel: w120 -> [w126 _]
              frame "Voltage Level " {
                n50 = property on="Ref Voltage level for Settling Time Calc" class="DigNum (strict)"(error in=w128, "Value"=w126) -> (error out=w127:errorcluster)  [unwired: 1 in, 1 out]
              }
              frame "Percentage of Vnom", Default {
              }
            }
          }
          event "Percentage of Vnom (%)": Value Change {
            # "#TODO\nDo this logic when executing the testw"
            n51 = event-data() -> ("NewVal"=w131:dbl)  [unwired: 1 in]
            n52 = local read "Test Inputs"() -> (w134:T10)
            n53 = Unbundle By Name(w134) -> ("Settling Time Calc Option"=w135:T11, "Nominal Output Voltage in V"=w130:dbl)
            n54 = case shown="\"Percentage of Vnom\"" w135 {
              tunnel: w132 -> [w137 w143]
              tunnel: [w137 w139] -> w133
              tunnel: w131 -> [_ w138]
              tunnel: w130 -> [_ w140]
              frame "Voltage Level ", Default {
              }
              frame "Percentage of Vnom" {
                n55 = formula code="y = (x/100)*v;"("v"=w140, "x"=w138) -> ("y"=w141:dbl)
                n56 = property on="Ref Voltage level for Settling Time Calc" class="DigNum (strict)"(error in=w143, "Value"=w141) -> (error out=w142:errorcluster)  [unwired: 1 in, 1 out]
                n57 = property on="% of Vnom for Settling Time Calc" class="DigNum (strict)"(error in=w142, "Value"=w138) -> (error out=w139:errorcluster)  [unwired: 1 in, 1 out]
              }
            }
          }
          event "Take Transient snapshot?": Value Change {
            n58 = event-data() -> ("NewVal"=w144:bool)  [unwired: 1 in]
            n59 = property on="Save Transient Graph?" class="Bool (strict)"(error in=w146, "Value"=w144) -> (error out=w145:errorcluster)  [unwired: 1 in, 1 out]
          }
          event "Save Scope Raw Data?": Value Change {
            n60 = event-data() -> ("NewVal"=w148:bool)  [unwired: 1 in]
            n61 = property on="Save Scope Raw Data?" class="Bool (strict)"(error in=w150, "Value"=w148) -> (error out=w149:errorcluster)  [unwired: 1 in, 1 out]
          }
          event "Auto Scale Y-Axis?": Value Change {
            n62 = event-data() -> ("NewVal"=w152:bool)  [unwired: 1 in]
            n63 = property on="Auto Scale Y-Axis?" class="Bool (strict)"(error in=w154, "Value"=w152) -> (error out=w153:errorcluster)  [unwired: 1 in, 1 out]
          }
          event "SystemSetup": Value Change {
            n64 = event-data() -> ("NewVal"=w161:T4)  [unwired: 1 in]
            n65 = Unbundle By Name(w161) -> ("Set Input Voltage.PinName"=w165:string, "Set Load Current.PinName"=w164:string, "Measure Output Voltage.PinName"=w163:string, "Measure Input Voltage.PinName"=w156:string)
            n66 = Bundle By Name(cluster=w162, "Test Pins.Set Input Voltage"=w165, "Test Pins.Set Load Current"=w164, "Test Pins.Measure Output Voltage"=w163, "Test Pins.Measure Input Voltage"=w156) -> (w158:T19)
            n67 = Unbundle By Name(w158) -> ("Test Pins"=w157:T9)
            n68 = property on="Test Pins" class="Clust (strict)"(error in=w159, "Value"=w157) -> (error out=w160:errorcluster)  [unwired: 1 in, 1 out]
          }
          event Value Change {
            n69 = event-data() -> ("NewVal"=w166:T9, "NewVal.Set Input Voltage"=w167:string, "NewVal.Set Load Current"=w172:string, "NewVal.Measure Output Voltage"=w171:string, "NewVal.Measure Input Voltage"=w168:string)  [unwired: 1 in]
            n70 = Bundle By Name(cluster=w173, "Test Pins"=w166) -> (w174:T19)
            n71 = property on="SystemSetup" class="Clust (strict)"(error in=w177) -> (error out=w170:errorcluster, "Value"=w169:T22)  [unwired: 1 in, 1 out]
            n72 = Bundle By Name(cluster=w169, "Set Vin.PinName"=w167, "Set Iload.PinName"=w172, "Capture Vout.PinName"=w171, "Capture Vin.PinName"=w168) -> (w175:T22)
            n73 = property on="SystemSetup" class="Clust (strict)"(error in=w170, "Value"=w175) -> (error out=w176:errorcluster)  [unwired: 1 in, 1 out]
          }
          event Value Change {
            n74 = event-data() -> ("NewVal.Advance Setting"=w213:T12, "NewVal.Input Voltage Vin1 in V"=w205:dbl, "NewVal.Input Voltage Vin2 in V"=w204:dbl, "NewVal.Duration of the pulse in s"=w181:dbl, "NewVal.Nominal Output Voltage in V"=w203:dbl, "NewVal.Ref Voltage level for Settling Time Calc"=w202:dbl, "NewVal.% of Vnom for Settling Time Calc"=w201:dbl, "NewVal.Settling Time Calc Option"=w200:T11, "NewVal.Save Transient Graph?"=w196:bool, "NewVal.Load Current in A"=w180:dbl, "NewVal.Save Scope Raw Data?"=w189:bool, "NewVal.Delay - t1 (s)"=w178:dbl, "NewVal.Delay - t2 (s)"=w179:dbl, "NewVal.Auto Scale Y-Axis?"=w188:bool)  [unwired: 1 in]
            n75 = property on="Take Transient snapshot?" class="Bool (strict)"(error in=w187, "Value"=w196) -> (error out=w197:errorcluster)  [unwired: 1 in, 1 out]
            n76 = property on="Input \nVoltage 1 \n- Vin1 (V)" class="DigNum (strict)"(error in=w187, "Value"=w205) -> (error out=w206:errorcluster)  [unwired: 1 in, 1 out]
            n77 = property on="Input \nVoltage 2 \n- Vin2 (V)" class="DigNum (strict)"(error in=w206, "Value"=w204) -> (error out=w207:errorcluster)  [unwired: 1 in, 1 out]
            n78 = property on="Load Current (A)" class="DigNum (strict)"(error in=w197, "Value"=w180) -> (error out=w195:errorcluster)  [unwired: 1 in, 1 out]
            n79 = property on="Duration of the pulse (s)" class="DigNum (strict)"(error in=w207, "Value"=w181) -> (error out=w208:errorcluster)  [unwired: 1 in, 1 out]
            n80 = property on="Save Scope Raw Data?" class="Bool (strict)"(error in=w195, "Value"=w189) -> (error out=w194:errorcluster)  [unwired: 1 in, 1 out]
            n81 = property on="Nominal Output Voltage (V)" class="DigNum (strict)"(error in=w208, "Value"=w203) -> (error out=w209:errorcluster)  [unwired: 1 in, 1 out]
            n82 = property on="Delay - t1 (s)" class="DigNum (strict)"(error in=w194, "Value"=w178) -> (error out=w193:errorcluster)  [unwired: 1 in, 1 out]
            n83 = property on="Delay - t2 (s)" class="DigNum (strict)"(error in=w193, "Value"=w179) -> (error out=w190:errorcluster)  [unwired: 1 in, 1 out]
            n84 = property on="Voltage to \nsettle above Vnom (V)" class="DigNum (strict)"(error in=w209, "Value"=w202) -> (error out=w210:errorcluster)  [unwired: 1 in, 1 out]
            n85 = Compound Arithmetic op=ADD(w181, w178, w179) -> (w186:dbl)
            n86 = property on="Auto Scale Y-Axis?" class="Bool (strict)"(error in=w190, "Value"=w188) -> (error out=w183:errorcluster)  [unwired: 1 in, 1 out]
            n87 = Bundle By Name(cluster=w211, "Test Inputs.Advance Setting"=w213) -> (w212:T19)
            n88 = property on="Percentage \nof Vnom (%)" class="DigNum (strict)"(error in=w210, "Value"=w201) -> (error out=w214:errorcluster)  [unwired: 1 in, 1 out]
            n89 = Multiply(x=w186, y=5.0) -> (x*y=w184:dbl)
            n90 = Type Cast(type=enum32{"Item 0", "Item 1"}."Item 0" ("Settling Time Calculation"), x=w200) -> (*(type *) &x=w198:enum32{"Item 0", "Item 1"})
            n91 = property on="Sequence Timeout" class="DigNum (strict)"(error in=w183, "Value"=w184) -> (error out=w182:errorcluster)  [unwired: 1 in, 1 out]
            n92 = property on="Settling Time Calculation" class="RadioBtnsControl (strict)"(error in=w214, "Value"=w198) -> (error out=w192:errorcluster)  [unwired: 1 in, 1 out]
            n93 = Merge Errors(w192, w182) -> (w191:errorcluster)
          }
          event "Tab Enum": Value Change {
            n94 = event-data() -> ("NewVal"=→"Tab Control":T1)  [unwired: 1 in]
          }
          event "Advanced Settings": Value Change {
            n95 = event-data() -> ()  [unwired: 1 in, 1 out]
            n96 = Unbundle By Name(w221) -> ("Test Inputs.Advance Setting"=w223:T12)
            n97 = call "Advance Settings UI.vi"("Advance Setting In"=w223, "error in (no error)"=w224) -> ("Advance Setting Out"=w218:T12, "error out"=w220:errorcluster)  [unwired: 12 in]
            n98 = Bundle By Name(cluster=w221, "Test Inputs.Advance Setting"=w218) -> (w222:T19)
            n99 = property on="Advance Setting" class="Clust (strict)"(error in=w220, "Value"=w218) -> (error out=w219:errorcluster)  [unwired: 1 in, 1 out]
          }
        }
      }
      frame "----------------- Macro ---------------" {
        # "Not used. category splitter"
      }
      frame "Macro: Initialize" {
        w233 = string[] ["Macro: GUI Start"]  # Standalone: Start the debug
        w234 = string[] ["Macro: Execute Test", "Exit"]  # Automation: Execute and stop
        # "Hidden in UI"
        # "This case decides the mode of the execution. Debug Mode: The plugin will act as a standalone GUI where user can change inputs, run test and debug the system. automation mode: The plugin will act as a flat code and go through all the test procedures and stops."
        n100 = call <userlib>:"Get Mode.vi"("Caller Information"="Caller Information", "error in (no error)"=w236) -> ("Automation(F) \\ Standalone (T)"=w232:bool, "error out"=w235:errorcluster)  [unwired: 12 in]
        n101 = Bundle By Name(cluster=w240, "Termination Monitor Info.Caller Information"="Caller Information") -> (w229:T19)
        n102 = Select(t=w233, s=w232, f=w234) -> (s? t:f=w231:string[])
        n103 = call <userlib>:"Enqueue.vi"("Queue in"=w238, "States"=w231, "Enqueue at Front?(F)"=TRUE, "error in (no error)"=w235) -> ("error out"=w239:errorcluster)  [unwired: 10 in, 1 out]
      }
      frame "Macro: Execute Test" {
        w243 = string[] ["TerminationMonitor: Start", "Test: Start", "Test: Prepare Source SMU", "Test: Prepare Load SMU", "Test: Prepare Scope", "Test: Generate Input Voltage Seq", "Test: Set Load Current", "Test: Calc Min Delay for Max. Ref Position", "Test: Capture Transient", "Test: Capture Waveform Params", "Test: Calculate Out. Voltage Threshold", "Test: Calculate Settling Time", "Test: Cleanup DCPower", "Test: Cleanup Scope", "Test: Update UI", "Test: End", "TerminationMonitor: Stop"]  # Test Procedure
        # "List the states required for the test procedure. This state will be called in both automation mode and standalone mode when requested to run the test.\nDont remove 'Test: Start' and 'Test: End'."
        n104 = call <userlib>:"Enqueue.vi"("Queue in"=w250, "States"=w243, "Enqueue at Front?(F)"=TRUE, "error in (no error)"=w251) -> ("error out"=w245:errorcluster)  [unwired: 10 in, 1 out]
        n105 = Array Size(array=w243) -> (size(s)=w242:i32)
        n106 = call "Progress Monitor.vi"("State Array []"=w243, "Option (Default: Get State Index)"=Progress_Monitor_Option."State Array Init" ("Option")) -> ()  [unwired: 13 in, 1 out]
        n107 = property on="Progress" class="Slide (strict)"(error in=w245, "Visible"=TRUE, "Scale.Maximum"=w242, "Value"=0 ("Progress")) -> (error out=w247:errorcluster)  [unwired: 1 in, 1 out]
      }
      frame "Macro: GUI Start" {
        # "Initialize the data cluster for the standalone mode and register for the event from caller.\nDon't remove 'GUI: Initialize Data' and 'GUI: Register Event'."
        n108 = call <userlib>:"Enqueue.vi"("Queue in"=w255, "States"=string[] ["GUI: Initialize Data", "GUI: Register Event"], "Enqueue at Front?(F)"=TRUE, "error in (no error)"=w257) -> ("error out"=w258:errorcluster)  [unwired: 10 in, 1 out]
      }
      frame "Macro: GUI Stop" {
        # "Cleanups the standalone mode and stop the execution.\nDon't remove 'GUI: Unregister Event', 'GUI: Cleanup Data' and 'Exit'."
        n109 = call <userlib>:"Enqueue.vi"("Queue in"=w262, "States"=string[] ["GUI: Unregister Event", "GUI: Cleanup Data", "Exit"], "Enqueue at Front?(F)"=TRUE, "error in (no error)"=w264) -> ("error out"=w265:errorcluster)  [unwired: 10 in, 1 out]
      }
      frame "--------------- GUI Mode-----------------" {
        # "Not used. category splitter"
      }
      frame "GUI: Initialize Data" {
        w295 = T23 {"Major Color"=14737632, "Minor Color"=15987699} ("Y Scale.Grid Colors")
        w303 = T24 {"relativeInitialX"=0.0, "xIncrement"=0.0, "wfm"=[]} ("Output Voltage Measured")
        w304 = dbl[] []  # Input Voltage Waveform
        w306 = T1."Station Setup" ("Tab Enum")
        w309 = string[][] []  # Test Results[][]
        w318 = T15 {"Output Voltage Measured"={"relativeInitialX"=0.0, "xIncrement"=0.0, "wfm"=[]}, "Input Voltage Measured"={"relativeInitialX"=0.0, "xIncrement"=0.0, "wfm"=[]}, "Actual Sample Rate"=0.0, "First Edge - Settling Time in s"=0.0, "Second Edge - Settling Time in s"=0.0}  # Test Results
        # "Add the front panel controls terminal here and connect them to the bundle structure, So they will be available through data cluster in every case. If the controls and indicators are added to the 'Test Inputs' & 'Test Results' cluster then they are already available in the data cluster since they are typedefs."
        n110 = local write "Tab Enum"(w306) -> ()
        n111 = local write "Tab Control"(w306) -> ()
        n112 = property on="Run" class="Bool (strict)"(error in=w312, "DisabledEnum"=T21."Enabled" ("Disabled")) -> (error out=w315:errorcluster)  [unwired: 1 in, 1 out]
        n113 = property on="Terminate" class="Bool (strict)"(error in=w315, "DisabledEnum"=T21."Disabled and Grayed Out" ("Disabled")) -> (error out=w311:errorcluster)  [unwired: 1 in, 1 out]
        n114 = property on="Progress" class="Slide (strict)"(error in=w311, "Visible"=FALSE) -> (error out=w302:errorcluster)  [unwired: 1 in, 1 out]
        n115 = control-ref of="Line Transient"() -> (w291:refnum<vi>)
        n116 = property on="Line Transient" class="WFGraph (strict)"(error in=w302, "Active Plot"=u32 0, "Plot.YScaleIdx"=u32 0 ("Plot.Y Scale Index"), "Active Plot"=u32 1, "Plot.YScaleIdx"=u32 1 ("Plot.Y Scale Index")) -> (error out=w293:errorcluster)  [unwired: 1 in, 1 out]
        n117 = Bundle By Name(cluster=w317, "Test Pins"="Test Pins", "Test Inputs"="Test Inputs", "Test Results"=w318, "Test Results[][]"=w309, "Logger Folder Path"="DataLogPath", "Input Voltage Waveform"=w304, "Test Results.Input Voltage Measured"=w303, "Test Results.Output Voltage Measured"=w303, "Min delay for Reference Position"=u32 0) -> (w290:T19)
        n118 = property class="WFGraph (strict)"(reference=w291, error in=w293, "ActYScl"=0 ("Active Y Scale"), "YScale.GridColors"=w295, "ActYScl"=1 ("Active Y Scale"), "YScale.GridColors"=w295) -> (error out=w292:errorcluster)  [unwired: 1 out]
        n119 = control-ref of="Tab Enum"() -> (w287:refnum<vi>)
        n120 = control-ref of="Settling Time Calculation"() -> (w279:refnum<vi>)
        n121 = control-ref of="Advanced Settings"() -> (w276:refnum<vi>)
        n122 = control-ref of="Auto Scale Y-Axis?"() -> (w275:refnum<vi>)
        n123 = control-ref of="Save Scope Raw Data?"() -> (w274:refnum<vi>)
        n124 = control-ref of="Take Transient snapshot?"() -> (w273:refnum<vi>)
        n125 = control-ref of="SystemSetup"() -> (w288:refnum<vi>)
        n126 = control-ref of="Input Voltage 1 - Vin1 (V)"() -> (w286:refnum<vi>)
        n127 = control-ref of="Input Voltage 2 - Vin2 (V)"() -> (w285:refnum<vi>)
        n128 = control-ref of="Load Current (A)"() -> (w284:refnum<vi>)
        n129 = control-ref of="Delay - t1 (s)"() -> (w283:refnum<vi>)
        n130 = control-ref of="Duration of the pulse (s)"() -> (w282:refnum<vi>)
        n131 = control-ref of="Delay - t2 (s)"() -> (w281:refnum<vi>)
        n132 = control-ref of="Nominal Output Voltage (V)"() -> (w280:refnum<vi>)
        n133 = control-ref of="Voltage to settle above Vnom (V)"() -> (w278:refnum<vi>)
        n134 = control-ref of="Percentage of Vnom (%)"() -> (w277:refnum<vi>)
        n135 = control-ref of="Second Edge - Settling Time (s)"() -> (w271:refnum<vi>)
        n136 = control-ref of="First Edge - Settling Time (s)"() -> (w270:refnum<vi>)
        n137 = Build Array(w288, w287, w286, w285, w284, w283, w282, w281, w280, w279, w278, w277, w276, w275, w274, w273, w271, w270) -> (w272:refnum<vi>[])
        n138 = Bundle By Name(cluster=w290, "UI Ctls"=w272) -> (w289:T19)
      }
      frame "GUI: Register Event" {
        # "Hidden in UI"
        # "Register for the events from caller."
        n139 = register-events(error in=w323, "Caller Events") -> (reference out=w320:refnum<event-registration>, error out=w321:errorcluster)  [unwired: 1 in]
      }
      frame "GUI: Unregister Event" {
        n140 = Unregister For Events(event registration refnum=w324, error in=w327) -> (error out=w325:errorcluster)
      }
      frame "GUI: Cleanup Data" {
        # "Cleanup the reference or other resources before exiting"
      }
      frame "GUI: Get Logger File Path" {
        n141 = Unbundle By Name(w331) -> ("Logger Folder Path"=w338:path)
        n142 = call <vilib>:"Check if File or Folder Exists.vi"("error in (no error)"=w334, "path"=w338) -> ("error out"=w337:errorcluster, "file or folder exists?"=w336:bool, "dup path"=w335:path)  [unwired: 7 in]
        n143 = case shown="True" w336 {
          tunnel: [w341 w350] -> w333
          tunnel: w337 -> [w341 w353]
          tunnel: w331 -> [w340 w357]
          tunnel: [w340 w356] -> w332
          tunnel: w335 -> [_ w352]
          frame False {
          }
          frame True {
            n144 = Strip Path(path=w352) -> (name=w344:string)  [unwired: 1 out]
            n145 = call "Get Unique Name.vi"() -> ("date"=w351:string, "Unique String"=w343:string)  [unwired: 14 in]
            n146 = Concatenate Strings(w344, w351) -> (w347:string)
            n147 = Concatenate Strings(w344, w343) -> (w342:string)
            n148 = Concatenate Strings(w347, "\\" ("string"), w342) -> (w354:string)
            n149 = Build Path(base path=w352, name or relative path=w354) -> (appended path=w349:path)
            n150 = call <vilib>:"Create Directory Recursive.vi"("error in (no error)"=w353, "directory"=w349) -> ("error out"=w350:errorcluster, "directory copy"=w346:path)  [unwired: 3 in, 1 out]
            n151 = Build Path(base path=w346, name or relative path=w342) -> (appended path=w345:path)
            n152 = Bundle By Name(cluster=w357, "Valid Logger Path?"=TRUE ("Valid Logger path?"), "Logger File Path"=w345) -> (w356:T19)
          }
        }
      }
      frame "GUI: Log" {
        n153 = Unbundle By Name(w365) -> ("Test Inputs.Save Scope Raw Data?"=w358:bool, "Valid Logger Path?"=w359:bool, "Test Inputs"=w361:T10, "Test Results"=w362:T15, "Logger File Path"=w360:path)
        n154 = case shown="True" w359 {
          tunnel: [w367 w373] -> w364
          tunnel: w363 -> [w367 w372]
          tunnel: w362 -> [_ w371]
          tunnel: w361 -> [_ w370]
          tunnel: w360 -> [_ w369]
          tunnel: w358 -> [_ w368]
          frame False {
          }
          frame True {
            n155 = call "Log Data.vi"("Test Inputs"=w370, "Save Scope Data?"=w368, "Test Results"=w371, "DataLogger File Path"=w369, "error in (no error)"=w372) -> ("error out"=w373:errorcluster)  [unwired: 10 in]
          }
        }
      }
      frame "GUI: Update Graph Scale" {
        w379 = u32 1 ("Active Plot")
        w380 = u32 0 ("Active Plot")
        n156 = Unbundle By Name(w382) -> ("Test Inputs.Auto Scale Y-Axis?"=w381:bool)
        n157 = control-ref of="Line Transient"() -> (w375:refnum<vi>)
        n158 = property on="Property Node" class="WFGraph (strict)"(reference=w375, error in=w378, "Active Plot"=w380, "Plot.YScaleIdx"=w380, "Active Plot"=w379, "Plot.YScaleIdx"=w379) -> (reference out=w374:refnum<vi>, error out=w377:errorcluster)
        n159 = case shown="True" w381 {
          tunnel: [w384 w387] -> w376
          tunnel: w377 -> [w384 w386]
          tunnel: w374 -> [_ w385]
          frame False {
          }
          frame True {
            n160 = call "Two Plot Graph Auto Scale.vi"("Two Plot Graph Ref In"=w385, "error in (no error)"=w386) -> ("error out"=w387:errorcluster)  [unwired: 12 in, 1 out]
          }
        }
      }
      frame "GUI: Log Waveform Snapshot" {
        n161 = Unbundle By Name(w388) -> ("Test Inputs.Save Transient Graph?"=w394:bool, "Valid Logger Path?"=w392:bool, "Logger File Path"=w391:path)
        n162 = And(x=w394, y=w392) -> (x .and. y?=w393:bool)
        n163 = case shown="True" w393 {
          tunnel: w389 -> [w396 w401]
          tunnel: [w396 w397] -> w390
          tunnel: w391 -> [_ w419]
          frame False {
          }
          frame True {
            w407 = T23 {"Major Color"=14737632, "Minor Color"=15987699} ("Y Scale.Grid Colors")
            w408 = T23 {"Major Color"=16777216, "Minor Color"=16777216} ("Y Scale.Grid Colors")
            n164 = control-ref of="Line Transient"() -> (w412:refnum<vi>)
            n165 = call "Defer Front Panel.vi"("Defer Front Panel?"=TRUE, "error in"=w401) -> ("error out"=w402:errorcluster)  [unwired: 13 in]
            n166 = Path To String(path=w419) -> (string=w421:string)
            n167 = property class="WFGraph (strict)"(reference=w412, error in=w402, "ActYScl"=0 ("Active Y Scale"), "YScale.GridColors"=w408, "ActYScl"=1 ("Active Y Scale"), "YScale.GridColors"=w408) -> (reference out=w411:refnum<vi>, error out=w413:errorcluster)
            n168 = Concatenate Strings(w421, "_Waveform" ("string"), ".bmp" ("format string")) -> (w422:string)
            n169 = String To Path(string=w422) -> (path=w420:path)
            n170 = invoke class="WFGraph (strict)" method="Export Image"(reference=w411, error in=w413, "FileType"=enum32{"BMP", "EPS", "EMF", "PICT"}."BMP" ("File Type"), "Target"=enum32{"File", "Clipboard"}."File", "Path"=w420, "HideGrid"=TRUE ("Hide Grid")) -> (reference out=w403:refnum<vi>, error out=w404:errorcluster)  [unwired: 2 in, 6 out]
            n171 = property class="WFGraph (strict)"(reference=w403, error in=w404, "ActYScl"=0 ("Active Y Scale"), "YScale.GridColors"=w407, "ActYScl"=1 ("Active Y Scale"), "YScale.GridColors"=w407) -> (error out=w398:errorcluster)  [unwired: 1 out]
            n172 = call "Defer Front Panel.vi"("Defer Front Panel?"=FALSE, "error in"=w398) -> ("error out"=w397:errorcluster)  [unwired: 13 in]
          }
        }
      }
      frame "GUI: Set Busy" {
        n173 = call "Progress Monitor.vi"("State"=w423) -> ("State Array Index"=w426:i32)  [unwired: 14 in]
        n174 = property on="Progress" class="Slide (strict)"(error in=w424, "Value"=w426) -> (error out=w425:errorcluster)  [unwired: 1 in, 1 out]
        n175 = Unbundle By Name(w427) -> ("UI Ctls"=w432:refnum<vi>[])
        n176 = for {
          tunnel: [w437] -> w433 mode=indexing
          tunnel: w425 -> [w438]
          tunnel: w432 -> [w436] mode=indexing
          tunnel: T21."Disabled and Grayed Out" ("Disabled") -> [w435]
          n177 = property class="Ctl"(reference=w436, error in=w438, "DisabledEnum"=w435) -> (error out=w437:errorcluster)  [unwired: 1 out]
        }
        n178 = Merge Errors(w433) -> (w430:errorcluster)
        n179 = call "Defer Front Panel.vi"("Defer Front Panel?"=TRUE, "error in"=w430) -> ("error out"=w428:errorcluster)  [unwired: 13 in]
      }
      frame "GUI: Unset Busy" {
        n180 = call "Progress Monitor.vi"("State"=w439) -> ("State Array Index"=w442:i32)  [unwired: 14 in]
        n181 = property on="Progress" class="Slide (strict)"(error in=w440, "Value"=w442) -> (error out=w441:errorcluster)  [unwired: 1 in, 1 out]
        n182 = Unbundle By Name(w443) -> ("UI Ctls"=w448:refnum<vi>[])
        n183 = for {
          tunnel: [w453] -> w449 mode=indexing
          tunnel: w441 -> [w454]
          tunnel: w448 -> [w452] mode=indexing
          tunnel: T21."Enabled" ("Disabled") -> [w451]
          n184 = property class="Ctl"(reference=w452, error in=w454, "DisabledEnum"=w451) -> (error out=w453:errorcluster)  [unwired: 1 out]
        }
        n185 = Merge Errors(w449) -> (w445:errorcluster)
        n186 = call "Defer Front Panel.vi"("Defer Front Panel?"=FALSE, "error in"=w445) -> ("error out"=w444:errorcluster)  [unwired: 13 in]
      }
      frame "GUI: Start Test" {
        n187 = property on="Run" class="Bool (strict)"(error in=w456, "DisabledEnum"=T21."Disabled and Grayed Out" ("Disabled")) -> (error out=w462:errorcluster)  [unwired: 1 in, 1 out]
        n188 = property on="Terminate" class="Bool (strict)"(error in=w462, "DisabledEnum"=T21."Enabled" ("Disabled")) -> (error out=w461:errorcluster)  [unwired: 1 in, 1 out]
        n189 = property on="Progress" class="Slide (strict)"(error in=w461, "Visible"=TRUE, "Value"=0 ("Progress")) -> (error out=w457:errorcluster)  [unwired: 1 in, 1 out]
      }
      frame "GUI: End Test" {
        n190 = property on="Run" class="Bool (strict)"(error in=w467, "Value"=FALSE ("Run"), "DisabledEnum"=T21."Enabled" ("Disabled")) -> (error out=w472:errorcluster)  [unwired: 1 in, 1 out]
        n191 = property on="Terminate" class="Bool (strict)"(error in=w472, "DisabledEnum"=T21."Disabled and Grayed Out" ("Disabled")) -> (error out=w470:errorcluster)  [unwired: 1 in, 1 out]
        n192 = property on="Progress" class="Slide (strict)"(error in=w470, "Visible"=FALSE) -> (error out=w468:errorcluster)  [unwired: 1 in, 1 out]
      }
      frame "GUI: Update Sequence Timeout" {
        # "Multiply by 5 to have sufficient timeout"
        n193 = Unbundle By Name(w477) -> ("Test Inputs.Delay - t1 (s)"=w483:dbl, "Test Inputs.Delay - t2 (s)"=w482:dbl, "Test Inputs.Duration of the pulse in s"=w481:dbl)
        n194 = Compound Arithmetic op=ADD(w483, w482, w481) -> (w478:dbl)
        n195 = Multiply(x=w478, y=5.0) -> (x*y=w480:dbl)
        n196 = property on="Sequence Timeout" class="DigNum (strict)"(error in=w476, "Value"=w480) -> (error out=w475:errorcluster)  [unwired: 1 in, 1 out]
      }
      frame "------------ TerminationMonitor -----------" {
        # "Not used. category splitter"
      }
      frame "TerminationMonitor: Start" {
        # "Termination Monitor monitors the execution of the caller. Use Termination Monitor Status to get the termination status. If the caller is terminating, stop the test procedure, cleanup and stop."
        n197 = Unbundle By Name(w490) -> ("Termination Monitor Info.Caller Information"=w489:T6)
        n198 = call <userlib>:"Termination Monitor Start.vi"("Caller Information"=w489, "error in (no error)"=w492) -> ("Termination Monitor Info out"=w488:T16, "error out"=w493:errorcluster)  [unwired: 12 in]
        n199 = Bundle By Name(cluster=w490, "Termination Monitor Info"=w488) -> (w491:T19)
      }
      frame "TerminationMonitor: Stop" {
        n200 = Unbundle By Name(w497) -> ("Termination Monitor Info"=w496:T16)
        n201 = call <userlib>:"Termination Monitor Stop.vi"("Status Info in"=w496, "error in (no error)"=w499) -> ("Status Info out"=w495:T16, "error out"=w500:errorcluster)  [unwired: 12 in]
        n202 = Bundle By Name(cluster=w497, "Termination Monitor Info"=w495) -> (w498:T19)
      }
      frame "------------ Automation Mode -----------" {
        # "Not used. category splitter"
      }
      frame "Test: Start" {
        # "Reinitialize/Reset/Update the data from the UI to the data cluster so that the data will be considered for the test procedure.\nReset the Test Results."
        n203 = call "Progress Monitor.vi"("State"=w508) -> ("State Array Index"=w505:i32)  [unwired: 14 in]
        n204 = property on="Progress" class="Slide (strict)"(error in=w506, "Value"=w505) -> (error out=w507:errorcluster)  [unwired: 1 in, 1 out]
        n205 = local read "DataLogPath"() -> (w510:path)
        n206 = local read "Test Inputs"() -> (w518:T10)
        n207 = local read "Test Pins"() -> (w511:T9)
        n208 = property on="Run" class="Bool (strict)"(error in=w507, "DisabledEnum"=T21."Disabled and Grayed Out" ("Disabled")) -> (error out=w514:errorcluster)  [unwired: 1 in, 1 out]
        n209 = Bundle By Name(cluster=w519, "Test Pins"=w511, "Test Inputs"=w518, "Test Results"=T15 {"Output Voltage Measured"={"relativeInitialX"=0.0, "xIncrement"=0.0, "wfm"=[]}, "Input Voltage Measured"={"relativeInitialX"=0.0, "xIncrement"=0.0, "wfm"=[]}, "Actual Sample Rate"=0.0, "First Edge - Settling Time in s"=0.0, "Second Edge - Settling Time in s"=0.0}, "Logger Folder Path"=w510) -> (w512:T19)
        n210 = property on="Terminate" class="Bool (strict)"(error in=w514, "DisabledEnum"=T21."Enabled" ("Disabled")) -> (error out=w509:errorcluster)  [unwired: 1 in, 1 out]
      }
      frame "Test: Prepare Source SMU" {
        w526 = 1025 items=["Automatically after Source Complete"=1025, "On Demand"=1026, "On Measure Trigger"=1027] ("Measurement:Advanced:Measure When")
        # "Doesn't turn off output"
        # "https://knowledge.ni.com/KnowledgeArticleDetails?id=kA00Z000000P6CsSAK&l=en-US"
        n211 = call "Progress Monitor.vi"("State"=w529) -> ("State Array Index"=w532:i32)  [unwired: 14 in]
        n212 = Unbundle By Name(w535) -> ("Test Pins.Set Input Voltage"=w521:string, "Test Inputs.Input Voltage Vin1 in V"=w525:dbl)
        n213 = property on="Progress" class="Slide (strict)"(error in=w530, "Value"=w532) -> (error out=w531:errorcluster)  [unwired: 1 in, 1 out]
        n214 = call "Prepare Source.vi"("Set Vin"=w521, "Initial Voltage Level (V)"=w525, "error in (no error)"=w531) -> ("error out"=w523:errorcluster)  [unwired: 12 in]
        n215 = call "Pin Name to Reference.vim"("Pin Name"=w521, "type"=refnum<k15> refnum ("instrument handle"), "error in (no error)"=w523) -> ("Reference"=w520:refnum<k15>, "error out"=w522:errorcluster)  [unwired: 7 in, 4 out]
        n216 = call <instrlib>:"niDCPower Abort With Channels.vi"("error in (no error)"=w522, "instrument handle"=w520) -> ("error out"=w528:errorcluster, "instrument handle out"=w527:refnum<k15>)  [unwired: 8 in]
        n217 = property class="niDCPower"(reference=w527, error in=w528, "Sequence Loop Count"=1 ("Source:Advanced:Sequence Loop Count"), "Measure When"=w526) -> (error out=w533:errorcluster)  [unwired: 1 out]
      }
      frame "Test: Prepare Load SMU" {
        n218 = call "Progress Monitor.vi"("State"=w541) -> ("State Array Index"=w544:i32)  [unwired: 14 in]
        n219 = property on="Progress" class="Slide (strict)"(error in=w542, "Value"=w544) -> (error out=w543:errorcluster)  [unwired: 1 in, 1 out]
        n220 = Unbundle By Name(w545) -> ("Test Pins.Set Load Current"=w539:string, "Test Inputs.Load Current in A"=w538:dbl, "Test Inputs.Advance Setting.Prepare.Load SMU Output Function"=w537:T14)
        n221 = call "Prepare Load.vi"("PinName"=w539, "Load Current Level (A)"=w538, "error in (no error)"=w543, "Load Output Function"=w537) -> ("error out"=w540:errorcluster)  [unwired: 11 in]
      }
      frame "Test: Prepare Scope" {
        # "Record Length = Sampling Rate x Acquired Time"
        # "Multiply by 2.5 to capture complete waveform including pretrigger"
        # "Abort the prev acquisition"
        n222 = Unbundle By Name(w555) -> ("Test Inputs.Duration of the pulse in s"=w559:dbl, "Test Inputs.Delay - t1 (s)"=w558:dbl, "Test Inputs.Delay - t2 (s)"=w557:dbl, "Test Pins.Measure Input Voltage"=w566:string, "Test Pins.Measure Output Voltage"=w547:string)
        n223 = call "Progress Monitor.vi"("State"=w574) -> ("State Array Index"=w577:i32)  [unwired: 14 in]
        n224 = property on="Progress" class="Slide (strict)"(error in=w575, "Value"=w577) -> (error out=w576:errorcluster)  [unwired: 1 in, 1 out]
        n225 = call "Pin Name to Reference.vim"("Pin Name"=w547, "type"=refnum<k15> refnum ("instrument handle"), "error in (no error)"=w576) -> ("Reference"=w552:refnum<k15>, "Channel"=w580:string, "error out"=w581:errorcluster)  [unwired: 7 in, 3 out]
        n226 = Compound Arithmetic op=ADD(w559, w558, w557) -> (w549:dbl)
        n227 = call <instrlib>:"niScope Abort.vi"("instrument handle"=w552, "error in"=w581) -> ("instrument handle out"=w551:refnum<k15>, "error out"=w553:errorcluster)  [unwired: 12 in]
        n228 = property class="niScope"(reference=w551, error in=w553, "Active Channel"=w580, "Channel Enabled"=TRUE ("Vertical:Channel Enabled")) -> (error out=w568:errorcluster, "Vertical Coupling"=w554:i32)  [unwired: 1 out]
        n229 = call "Pin Name to Reference.vim"("Pin Name"=w566, "type"=refnum<k15> refnum ("instrument handle"), "error in (no error)"=w568) -> ("Reference"=w571:refnum<k15>, "Channel"=w570:string, "error out"=w572:errorcluster)  [unwired: 7 in, 3 out]
        n230 = property class="niScope"(reference=w571, error in=w572, "Active Channel"=w570, "Channel Enabled"=TRUE ("Vertical:Channel Enabled")) -> (reference out=w564:refnum<k15>, error out=w567:errorcluster)
        n231 = Multiply(x=w549, y=2.5) -> (x*y=w548:dbl)
        n232 = property class="niScope"(reference=w564, error in=w567) -> (reference out=w562:refnum<k15>, error out=w565:errorcluster, "Actual Sample Rate"=w560:dbl)
        n233 = Multiply(x=w548, y=w560) -> (x*y=w578:dbl)
        n234 = To Long Integer(number=w578) -> (32bit integer=w561:i32)
        n235 = property class="niScope"(reference=w562, error in=w565, "Min Number of Points"=w561, "Min Sample Rate"=w560) -> (error out=w563:errorcluster)  [unwired: 1 out]
        n236 = Bundle By Name(cluster=w555, "Output Voltage Coupling"=w554) -> (w556:T19)
      }
      frame "Test: Generate Input Voltage Seq" {
        n237 = Unbundle By Name(w592) -> ("Test Inputs.Input Voltage Vin1 in V"=w585:dbl, "Test Inputs.Input Voltage Vin2 in V"=w596:dbl, "Test Inputs.Delay - t1 (s)"=w587:dbl, "Test Inputs.Delay - t2 (s)"=w586:dbl, "Test Inputs.Duration of the pulse in s"=w595:dbl)
        n238 = call "Progress Monitor.vi"("State"=w588) -> ("State Array Index"=w591:i32)  [unwired: 14 in]
        n239 = property on="Progress" class="Slide (strict)"(error in=w589, "Value"=w591) -> (error out=w590:errorcluster)  [unwired: 1 in, 1 out]
        n240 = Build Array(w585, w596, w585) -> (w594:dbl[])
        n241 = Build Array(w587, w595, w586) -> (w584:dbl[])
        n242 = Bundle By Name(cluster=w592, "Input Voltage Waveform"=w594, "Input Voltage Source Delay"=w584) -> (w593:T19)
      }
      frame "Test: Set Load Current" {
        w608 = T25 1030 items=["Source Complete Event"=1030, "Measure Complete Event"=1031, "Sequence Iteration Complete Event"=1032, "Sequence Engine Done Event"=1033, "Pulse Complete Event"=1051, "Ready For Pulse Trigger Event"=1052] ("event")
        n243 = call "Progress Monitor.vi"("State"=w598) -> ("State Array Index"=w601:i32)  [unwired: 14 in]
        n244 = property on="Progress" class="Slide (strict)"(error in=w599, "Value"=w601) -> (error out=w600:errorcluster)  [unwired: 1 in, 1 out]
        n245 = Unbundle By Name(w606) -> ("Test Inputs.Load Current in A"=w603:dbl, "Test Pins.Set Load Current"=w605:string)
        n246 = Absolute Value(x=w603) -> (abs(x)=w604:dbl)
        n247 = Negate(x=w604) -> (-x=w602:dbl)
        n248 = call "Pin Name to Reference.vim"("Pin Name"=w605, "type"=refnum<k15> refnum ("instrument handle"), "error in (no error)"=w600) -> ("Reference"=w611:refnum<k15>, "error out"=w613:errorcluster)  [unwired: 7 in, 4 out]
        n249 = call <instrlib>:"niDCPower Configure Current Level.vi"("error in (no error)"=w613, "current level"=w602, "instrument handle"=w611) -> ("error out"=w610:errorcluster, "instrument handle out"=w609:refnum<k15>)  [unwired: 7 in]
        n250 = call <instrlib>:"niDCPower Wait For Event With Channels.vi"("error in (no error)"=w610, "event"=w608, "instrument handle"=w609) -> ("error out"=w607:errorcluster)  [unwired: 7 in, 1 out]
      }
      frame "Test: Calc Min Delay for Max. Ref Position" {
        # "in milliseconds"
        # "Total Acquisition Length"
        n251 = Unbundle By Name(w623) -> ("Test Pins.Measure Input Voltage"=w633:string)
        n252 = call "Progress Monitor.vi"("State"=w615) -> ("State Array Index"=w618:i32)  [unwired: 14 in]
        n253 = property on="Progress" class="Slide (strict)"(error in=w616, "Value"=w618) -> (error out=w617:errorcluster)  [unwired: 1 in, 1 out]
        n254 = call "Pin Name to Reference.vim"("Pin Name"=w633, "type"=refnum<k15> refnum ("instrument handle"), "error in (no error)"=w617) -> ("Reference"=w635:refnum<k15>, "error out"=w636:errorcluster)  [unwired: 7 in, 4 out]
        n255 = property class="niScope"(reference=w635, error in=w636) -> (error out=w634:errorcluster, "Reference Position"=w619:dbl, "Min Number of Points"=w620:i32, "Actual Sample Rate"=w632:dbl)  [unwired: 1 out]
        n256 = Reciprocal(x=w632) -> (1/x=w631:dbl)
        n257 = To Double Precision Float(number=w620) -> (double precision float=w630:dbl)
        n258 = Multiply(x=w630, y=w631) -> (x*y=w629:dbl)
        n259 = Divide(x=w619, y=100.0) -> (x/y=w628:dbl)
        n260 = Multiply(x=w628, y=w629) -> (x*y=w626:dbl)
        n261 = Multiply(x=w626, y=1000.0) -> (x*y=w622:dbl)
        n262 = To Unsigned Long Integer(number=w622) -> (unsigned 32bit integer=w621:u32)
        n263 = Bundle By Name(cluster=w623, "Min delay for Reference Position"=w621) -> (w624:T19)
      }
      frame "Test: Capture Transient" {
        w656 = T25 1033 items=["Source Complete Event"=1030, "Measure Complete Event"=1031, "Sequence Iteration Complete Event"=1032, "Sequence Engine Done Event"=1033, "Pulse Complete Event"=1051, "Ready For Pulse Trigger Event"=1052] ("event")
        w682 = T26 1006 items=["DC Voltage"=1006, "DC Current"=1007, "Pulse Voltage"=1049, "Pulse Current"=1050] ("output function")
        w683 = T27 1021 items=["Single Point"=1020, "Sequence"=1021] ("source mode")
        # "Multiply timeout with 5 for smu and scopeto ensure timeout is large enough"
        # "#TODO Split this into 3 cases\n\nStart Scope Acquisition\nSet SMU Voltage Sequence\nScope Capture"
        n264 = Unbundle By Name(w686) -> ("Input Voltage Source Delay"=w642:dbl[], "Test Pins.Set Input Voltage"=w688:string, "Input Voltage Waveform"=w691:dbl[], "Min delay for Reference Position"=w663:u32, "Test Pins.Measure Input Voltage"=w655:string, "Test Pins.Measure Output Voltage"=w654:string)
        n265 = call "Progress Monitor.vi"("State"=w673) -> ("State Array Index"=w676:i32)  [unwired: 14 in]
        n266 = property on="Progress" class="Slide (strict)"(error in=w674, "Value"=w676) -> (error out=w675:errorcluster)  [unwired: 1 in, 1 out]
        n267 = call "Pin Name to Reference.vim"("Pin Name"=w654, "type"=refnum<k15> refnum ("instrument handle"), "error in (no error)"=w675) -> ("Reference"=w690:refnum<k15>, "Channel"=w653:string, "error out"=w669:errorcluster)  [unwired: 7 in, 3 out]
        n268 = call "Pin Name to Reference.vim"("Pin Name"=w655, "type"=refnum<k15> refnum ("instrument handle"), "error in (no error)"=w669) -> ("Channel"=w667:string, "error out"=w668:errorcluster)  [unwired: 7 in, 4 out]
        n269 = call <instrlib>:"niScope Initiate Acquisition.vi"("instrument handle"=w690, "error in"=w668) -> ("instrument handle out"=w648:refnum<k15>, "error out"=w662:errorcluster)  [unwired: 12 in]
        n270 = Build Array(w667, w653) -> (w666:string[])
        n271 = flat-sequence {
          tunnel: w663 -> [w700]
          tunnel: w662 -> [w699]
          tunnel: [w699] -> w645
          frame #0 {
            n272 = Wait (ms)(milliseconds to wait=w700) -> ()  [unwired: 1 out]
          }
        }
        n273 = Array To Spreadsheet String(delimiter (Tab)=",", array=w666, 3:"" ("format string")) -> (spreadsheet string=w660:string)
        n274 = property class="niScope"(reference=w648, error in=w645) -> (reference out=w647:refnum<k15>, error out=w646:errorcluster, "Actual Record Length"=w652:i32, "Actual Sample Rate"=w644:dbl)
        n275 = call "Pin Name to Reference.vim"("Pin Name"=w688, "type"=refnum<k15> refnum ("instrument handle"), "error in (no error)"=w645) -> ("Reference"=w678:refnum<k15>, "error out"=w680:errorcluster)  [unwired: 7 in, 4 out]
        n276 = call <instrlib>:"niDCPower Configure Source Mode With Channels.vi"("error in (no error)"=w680, "source mode"=w683, "instrument handle"=w678) -> ("error out"=w684:errorcluster, "instrument handle out"=w681:refnum<k15>)  [unwired: 7 in]
        n277 = call <instrlib>:"niDCPower Configure Output Function.vi"("error in (no error)"=w684, "output function"=w682, "instrument handle"=w681) -> ("error out"=w679:errorcluster, "instrument handle out"=w677:refnum<k15>)  [unwired: 7 in]
        n278 = To Double Precision Float(number=w652) -> (double precision float=w651:dbl)
        n279 = Divide(x=w651, y=w644) -> (x/y=w650:dbl)
        n280 = call <instrlib>:"niDCPower Set Sequence.vi"("source delays"=w642, "error in (no error)"=w679, "values"=w691, "instrument handle"=w677) -> ("error out"=w695:errorcluster, "instrument handle out"=w694:refnum<k15>)  [unwired: 1 in, 5 out]
        n281 = Add Array Elements(numeric array=w642) -> (sum=w641:dbl)
        n282 = Multiply(x=5.0, y=w650) -> (x*y=w643:dbl)
        n283 = call <instrlib>:"niDCPower Commit With Channels.vi"("error in (no error)"=w695, "instrument handle"=w694) -> ("error out"=w693:errorcluster, "instrument handle out"=w692:refnum<k15>)  [unwired: 8 in]
        n284 = call <instrlib>:"niDCPower Initiate With Channels.vi"("error in (no error)"=w693, "instrument handle"=w692) -> ("error out"=w659:errorcluster, "instrument handle out"=w657:refnum<k15>)  [unwired: 8 in]
        n285 = Multiply(x=w641, y=5.0) -> (x*y=w639:dbl)
        n286 = call-poly <instrlib>:"niScope Fetch (poly).vi"("timeout"=w643, "error in"=w646, "channels"=w660, "instrument handle"=w647) -> ("error out"=w661:errorcluster, "waveform"=w685:T5)  [unwired: 4 in, 2 out]
        n287 = call <instrlib>:"niDCPower Wait For Event With Channels.vi"("timeout (sec)"=w639, "error in (no error)"=w659, "event"=w656, "instrument handle"=w657) -> ("error out"=w658:errorcluster)  [unwired: 6 in, 1 out]
        n288 = Index Array(array=w685) -> (element #1=w672:T24, element #2=w671:T24)  [unwired: 2 in]
        n289 = Merge Errors(w658, w661) -> (w689:errorcluster)
        n290 = Bundle By Name(cluster=w686, "Test Results.Input Voltage Measured"=w672, "Test Results.Output Voltage Measured"=w671, "Test Results.Actual Sample Rate"=w644) -> (w687:T19)
      }
      frame "Test: Capture Waveform Params" {
        w712 = T28 7 items=["None"=4000, "Frequency"=2, "Average Frequency"=1016, "FFT Frequency"=1008, "Period"=3, "Average Period"=1015, "Rise Time"=0, "Fall Time"=1, "Rising Slew Rate"=1010, "Falling Slew Rate"=1011, "Overshoot"=18, "Preshoot"=19, "Voltage RMS"=4, "Voltage Cycle RMS"=16, "AC Estimate"=1012, "FFT Amplitude"=1009, "Voltage Average"=10, "Voltage Cycle Average"=17, "DC Estimate"=1013, "Voltage Max"=6, "Voltage Min"=7, "Voltage Peak-to-Peak"=5, "Voltage High"=8, "Voltage Low"=9, "Voltage Amplitude"=15, "Voltage Top"=1007, "Voltage Base"=1006, "Voltage Base-to-Top"=1017, "Negative Width"=11, "Positive Width"=12, "Negative Duty Cycle"=13, "Positive Duty Cycle"=14, "Integral"=1005, "Area"=1003, "Cycle Area"=1004, "Time Delay"=1014, "Phase Delay"=1018, "Low Ref Volts"=1000, "Mid Ref Volts"=1001, "High Ref Volts"=1002, "Volt. Hist. Mean"=2000, "Volt. Hist. Stdev"=2001, "Volt. Hist. Median"=2003, "Volt. Hist. Mode"=2010, "Volt. Hist. Max"=2005, "Volt. Hist. Min"=2006, "Volt. Hist. Peak-to-Peak"=2002, "Volt. Hist. Mean + Stdev"=2007, "Volt. Hist. Mean + 2 Stdev"=2008, "Volt. Hist. Mean + 3 Stdev"=2009, "Volt. Hist. Hits"=2004, "Volt. Hist. New Hits"=2011, "Time Hist. Mean"=3000, "Time Hist. Stdev"=3001, "Time Hist. Median"=3003, "Time Hist. Mode"=3010, "Time Hist. Max"=3005, "Time Hist. Min"=3006, "Time Hist. Peak-to-Peak"=3002, "Time Hist. Mean + Stdev"=3007, "Time Hist. Mean + 2 Stdev"=3008, "Time Hist. Mean + 3 Stdev"=3009, "Time Hist. Hits"=3004, "Time Hist. New Hits"=3011] ("scalar measurement")
        w714 = T28 6 items=["None"=4000, "Frequency"=2, "Average Frequency"=1016, "FFT Frequency"=1008, "Period"=3, "Average Period"=1015, "Rise Time"=0, "Fall Time"=1, "Rising Slew Rate"=1010, "Falling Slew Rate"=1011, "Overshoot"=18, "Preshoot"=19, "Voltage RMS"=4, "Voltage Cycle RMS"=16, "AC Estimate"=1012, "FFT Amplitude"=1009, "Voltage Average"=10, "Voltage Cycle Average"=17, "DC Estimate"=1013, "Voltage Max"=6, "Voltage Min"=7, "Voltage Peak-to-Peak"=5, "Voltage High"=8, "Voltage Low"=9, "Voltage Amplitude"=15, "Voltage Top"=1007, "Voltage Base"=1006, "Voltage Base-to-Top"=1017, "Negative Width"=11, "Positive Width"=12, "Negative Duty Cycle"=13, "Positive Duty Cycle"=14, "Integral"=1005, "Area"=1003, "Cycle Area"=1004, "Time Delay"=1014, "Phase Delay"=1018, "Low Ref Volts"=1000, "Mid Ref Volts"=1001, "High Ref Volts"=1002, "Volt. Hist. Mean"=2000, "Volt. Hist. Stdev"=2001, "Volt. Hist. Median"=2003, "Volt. Hist. Mode"=2010, "Volt. Hist. Max"=2005, "Volt. Hist. Min"=2006, "Volt. Hist. Peak-to-Peak"=2002, "Volt. Hist. Mean + Stdev"=2007, "Volt. Hist. Mean + 2 Stdev"=2008, "Volt. Hist. Mean + 3 Stdev"=2009, "Volt. Hist. Hits"=2004, "Volt. Hist. New Hits"=2011, "Time Hist. Mean"=3000, "Time Hist. Stdev"=3001, "Time Hist. Median"=3003, "Time Hist. Mode"=3010, "Time Hist. Max"=3005, "Time Hist. Min"=3006, "Time Hist. Peak-to-Peak"=3002, "Time Hist. Mean + Stdev"=3007, "Time Hist. Mean + 2 Stdev"=3008, "Time Hist. Mean + 3 Stdev"=3009, "Time Hist. Hits"=3004, "Time Hist. New Hits"=3011] ("scalar measurement")
        w723 = T28 7 items=["None"=4000, "Frequency"=2, "Average Frequency"=1016, "FFT Frequency"=1008, "Period"=3, "Average Period"=1015, "Rise Time"=0, "Fall Time"=1, "Rising Slew Rate"=1010, "Falling Slew Rate"=1011, "Overshoot"=18, "Preshoot"=19, "Voltage RMS"=4, "Voltage Cycle RMS"=16, "AC Estimate"=1012, "FFT Amplitude"=1009, "Voltage Average"=10, "Voltage Cycle Average"=17, "DC Estimate"=1013, "Voltage Max"=6, "Voltage Min"=7, "Voltage Peak-to-Peak"=5, "Voltage High"=8, "Voltage Low"=9, "Voltage Amplitude"=15, "Voltage Top"=1007, "Voltage Base"=1006, "Voltage Base-to-Top"=1017, "Negative Width"=11, "Positive Width"=12, "Negative Duty Cycle"=13, "Positive Duty Cycle"=14, "Integral"=1005, "Area"=1003, "Cycle Area"=1004, "Time Delay"=1014, "Phase Delay"=1018, "Low Ref Volts"=1000, "Mid Ref Volts"=1001, "High Ref Volts"=1002, "Volt. Hist. Mean"=2000, "Volt. Hist. Stdev"=2001, "Volt. Hist. Median"=2003, "Volt. Hist. Mode"=2010, "Volt. Hist. Max"=2005, "Volt. Hist. Min"=2006, "Volt. Hist. Peak-to-Peak"=2002, "Volt. Hist. Mean + Stdev"=2007, "Volt. Hist. Mean + 2 Stdev"=2008, "Volt. Hist. Mean + 3 Stdev"=2009, "Volt. Hist. Hits"=2004, "Volt. Hist. New Hits"=2011, "Time Hist. Mean"=3000, "Time Hist. Stdev"=3001, "Time Hist. Median"=3003, "Time Hist. Mode"=3010, "Time Hist. Max"=3005, "Time Hist. Min"=3006, "Time Hist. Peak-to-Peak"=3002, "Time Hist. Mean + Stdev"=3007, "Time Hist. Mean + 2 Stdev"=3008, "Time Hist. Mean + 3 Stdev"=3009, "Time Hist. Hits"=3004, "Time Hist. New Hits"=3011] ("scalar measurement")
        w726 = T28 6 items=["None"=4000, "Frequency"=2, "Average Frequency"=1016, "FFT Frequency"=1008, "Period"=3, "Average Period"=1015, "Rise Time"=0, "Fall Time"=1, "Rising Slew Rate"=1010, "Falling Slew Rate"=1011, "Overshoot"=18, "Preshoot"=19, "Voltage RMS"=4, "Voltage Cycle RMS"=16, "AC Estimate"=1012, "FFT Amplitude"=1009, "Voltage Average"=10, "Voltage Cycle Average"=17, "DC Estimate"=1013, "Voltage Max"=6, "Voltage Min"=7, "Voltage Peak-to-Peak"=5, "Voltage High"=8, "Voltage Low"=9, "Voltage Amplitude"=15, "Voltage Top"=1007, "Voltage Base"=1006, "Voltage Base-to-Top"=1017, "Negative Width"=11, "Positive Width"=12, "Negative Duty Cycle"=13, "Positive Duty Cycle"=14, "Integral"=1005, "Area"=1003, "Cycle Area"=1004, "Time Delay"=1014, "Phase Delay"=1018, "Low Ref Volts"=1000, "Mid Ref Volts"=1001, "High Ref Volts"=1002, "Volt. Hist. Mean"=2000, "Volt. Hist. Stdev"=2001, "Volt. Hist. Median"=2003, "Volt. Hist. Mode"=2010, "Volt. Hist. Max"=2005, "Volt. Hist. Min"=2006, "Volt. Hist. Peak-to-Peak"=2002, "Volt. Hist. Mean + Stdev"=2007, "Volt. Hist. Mean + 2 Stdev"=2008, "Volt. Hist. Mean + 3 Stdev"=2009, "Volt. Hist. Hits"=2004, "Volt. Hist. New Hits"=2011, "Time Hist. Mean"=3000, "Time Hist. Stdev"=3001, "Time Hist. Median"=3003, "Time Hist. Mode"=3010, "Time Hist. Max"=3005, "Time Hist. Min"=3006, "Time Hist. Peak-to-Peak"=3002, "Time Hist. Mean + Stdev"=3007, "Time Hist. Mean + 2 Stdev"=3008, "Time Hist. Mean + 3 Stdev"=3009, "Time Hist. Hits"=3004, "Time Hist. New Hits"=3011] ("scalar measurement")
        n291 = Unbundle By Name(w717) -> ("Test Pins.Measure Input Voltage"=w727:string, "Test Pins.Measure Output Voltage"=w728:string)
        n292 = call "Progress Monitor.vi"("State"=w701) -> ("State Array Index"=w704:i32)  [unwired: 14 in]
        n293 = property on="Progress" class="Slide (strict)"(error in=w702, "Value"=w704) -> (error out=w703:errorcluster)  [unwired: 1 in, 1 out]
        n294 = call "Pin Name to Reference.vim"("Pin Name"=w728, "type"=refnum<k15> refnum ("instrument handle"), "error in (no error)"=w703) -> ("Reference"=w709:refnum<k15>, "Channel"=w707:string, "error out"=w711:errorcluster)  [unwired: 7 in, 3 out]
        n295 = call-poly <instrlib>:"niScope Fetch Measurement (poly).vi"("instrument handle"=w709, "channels"=w707, "scalar measurement"=w714, "error in"=w711) -> ("instrument handle out"=w708:refnum<k15>, "result"=w706:dbl, "error out"=w713:errorcluster)  [unwired: 9 in]
        n296 = call-poly <instrlib>:"niScope Fetch Measurement (poly).vi"("instrument handle"=w708, "channels"=w707, "scalar measurement"=w712, "error in"=w713) -> ("result"=w705:dbl, "error out"=w710:errorcluster)  [unwired: 9 in, 1 out]
        n297 = call "Pin Name to Reference.vim"("Pin Name"=w727, "type"=refnum<k15> refnum ("instrument handle"), "error in (no error)"=w710) -> ("Reference"=w720:refnum<k15>, "Channel"=w719:string, "error out"=w722:errorcluster)  [unwired: 7 in, 3 out]
        n298 = call-poly <instrlib>:"niScope Fetch Measurement (poly).vi"("instrument handle"=w720, "channels"=w719, "scalar measurement"=w726, "error in"=w722) -> ("instrument handle out"=w724:refnum<k15>, "result"=w716:dbl, "error out"=w725:errorcluster)  [unwired: 9 in]
        n299 = call-poly <instrlib>:"niScope Fetch Measurement (poly).vi"("instrument handle"=w724, "channels"=w719, "scalar measurement"=w723, "error in"=w725) -> ("result"=w715:dbl, "error out"=w721:errorcluster)  [unwired: 9 in, 1 out]
        n300 = Bundle By Name(cluster=w717, "Output Voltage Params.Vmax"=w706, "Output Voltage Params.Vmin"=w705, "Output Voltage Params.Vmax"=w716, "Output Voltage Params.Vmin"=w715) -> (w718:T19)
      }
      frame "Test: Calculate Out. Voltage Threshold" {
        n301 = call "Progress Monitor.vi"("State"=w732) -> ("State Array Index"=w735:i32)  [unwired: 14 in]
        n302 = property on="Progress" class="Slide (strict)"(error in=w733, "Value"=w735) -> (error out=w734:errorcluster)  [unwired: 1 in, 1 out]
        n303 = Unbundle By Name(w736) -> ("Test Inputs.Settling Time Calc Option"=w742:T11, "Test Inputs.Ref Voltage level for Settling Time Calc"=w741:dbl, "Test Inputs.% of Vnom for Settling Time Calc"=w740:dbl, "Test Inputs.Nominal Output Voltage in V"=w739:dbl)
        n304 = case shown="\"Percentage of Vnom\"" w742 {
          tunnel: w741 -> [w744 _]
          tunnel: w740 -> [_ w746]
          tunnel: w739 -> [_ w747]
          tunnel: [w744 w745] -> w738
          frame "Voltage Level ", Default {
          }
          frame "Percentage of Vnom" {
            n305 = formula code="y = (x/100)*v;"("x"=w746, "v"=w747) -> ("y"=w745:dbl)
          }
        }
        n306 = Bundle By Name(cluster=w736, "Test Inputs.Ref Voltage level for Settling Time Calc"=w738) -> (w737:T19)
      }
      frame "Test: Calculate Settling Time" {
        n307 = call "Progress Monitor.vi"("State"=w756) -> ("State Array Index"=w759:i32)  [unwired: 14 in]
        n308 = Unbundle By Name(w760) -> ("Output Voltage Coupling"=w748:i32, "Test Results.Output Voltage Measured.wfm"=w755:dbl[], "Test Inputs.Ref Voltage level for Settling Time Calc"=w754:dbl, "Test Inputs.Duration of the pulse in s"=w753:dbl, "Test Results.Actual Sample Rate"=w752:dbl, "Test Inputs.Nominal Output Voltage in V"=w749:dbl)
        n309 = property on="Progress" class="Slide (strict)"(error in=w757, "Value"=w759) -> (error out=w758:errorcluster)  [unwired: 1 in, 1 out]
        n310 = call "CalculateSettlingTime.vi"("Waveform"=w755, "Waveform Coupling"=w748, "Recovery Volt Level (V)"=w754, "Duration of the pulse (s)"=w753, "Sampling Freq (S/s)"=w752, "DC Component (v)"=w749) -> ("FirstSpike. Duration (s)"=w751:dbl, "SecondSpike. Duration (s)"=w750:dbl)  [unwired: 8 in]
        n311 = Bundle By Name(cluster=w760, "Test Results.First Edge - Settling Time in s"=w751, "Test Results.Second Edge - Settling Time in s"=w750) -> (w761:T19)
      }
      frame "Test: Cleanup DCPower" {
        w763 = T27 1020 items=["Single Point"=1020, "Sequence"=1021] ("source mode")
        w770 = 1026 items=["Automatically after Source Complete"=1025, "On Demand"=1026, "On Measure Trigger"=1027] ("Measurement:Advanced:Measure When")
        w776 = T26 1006 items=["DC Voltage"=1006, "DC Current"=1007, "Pulse Voltage"=1049, "Pulse Current"=1050] ("output function")
        # "Default configuration"
        # "Resetting to DC Voltage mode because\nimport of soft panel config with voltage\nsequence mode throws error - Need to \ndebug further\n\nThis is a temporary fix"
        n312 = Unbundle By Name(w792) -> ("Test Pins.Set Input Voltage"=w788:string, "Test Pins.Set Load Current"=w790:string)
        n313 = call "Progress Monitor.vi"("State"=w777) -> ("State Array Index"=w780:i32)  [unwired: 14 in]
        n314 = property on="Progress" class="Slide (strict)"(error in=w778, "Value"=w780) -> (error out=w779:errorcluster)  [unwired: 1 in, 1 out]
        n315 = call "Pin Name to Reference.vim"("Pin Name"=w790, "type"=refnum<k15> refnum ("instrument handle"), "error in (no error)"=w779) -> ("Reference"=w783:refnum<k15>, "error out"=w784:errorcluster)  [unwired: 7 in, 4 out]
        n316 = call <instrlib>:"niDCPower Configure Output Enabled.vi"("error in (no error)"=w784, "output enabled"=FALSE, "instrument handle"=w783) -> ("error out"=w785:errorcluster, "instrument handle out"=w781:refnum<k15>)  [unwired: 7 in]
        n317 = call <instrlib>:"niDCPower Abort With Channels.vi"("error in (no error)"=w785, "instrument handle"=w781) -> ("error out"=w782:errorcluster)  [unwired: 8 in, 1 out]
        n318 = call "Pin Name to Reference.vim"("Pin Name"=w788, "type"=refnum<k15> refnum ("instrument handle"), "error in (no error)"=w782) -> ("Reference"=w787:refnum<k15>, "error out"=w786:errorcluster)  [unwired: 7 in, 4 out]
        n319 = call <instrlib>:"niDCPower Configure Output Enabled.vi"("error in (no error)"=w786, "output enabled"=FALSE, "instrument handle"=w787) -> ("error out"=w775:errorcluster, "instrument handle out"=w774:refnum<k15>)  [unwired: 7 in]
        n320 = call <instrlib>:"niDCPower Abort With Channels.vi"("error in (no error)"=w775, "instrument handle"=w774) -> ("error out"=w765:errorcluster, "instrument handle out"=w767:refnum<k15>)  [unwired: 8 in]
        n321 = call <instrlib>:"niDCPower Configure Source Mode With Channels.vi"("error in (no error)"=w765, "source mode"=w763, "instrument handle"=w767) -> ("error out"=w764:errorcluster, "instrument handle out"=w766:refnum<k15>)  [unwired: 7 in]
        n322 = call <instrlib>:"niDCPower Configure Output Function.vi"("error in (no error)"=w764, "output function"=w776, "instrument handle"=w766) -> ("error out"=w773:errorcluster, "instrument handle out"=w771:refnum<k15>)  [unwired: 7 in]
        n323 = property class="niDCPower"(reference=w771, error in=w773, "Measure When"=w770) -> (error out=w772:errorcluster)  [unwired: 1 out]
      }
      frame "Test: Cleanup Scope" {
        n324 = Unbundle By Name(w811) -> ("Test Pins.Measure Input Voltage"=w794:string, "Test Pins.Measure Output Voltage"=w810:string)
        n325 = call "Progress Monitor.vi"("State"=w806) -> ("State Array Index"=w809:i32)  [unwired: 14 in]
        n326 = property on="Progress" class="Slide (strict)"(error in=w807, "Value"=w809) -> (error out=w808:errorcluster)  [unwired: 1 in, 1 out]
        n327 = call "Pin Name to Reference.vim"("Pin Name"=w810, "type"=refnum<k15> refnum ("instrument handle"), "error in (no error)"=w808) -> ("Reference"=w814:refnum<k15>, "Channel"=w813:string, "error out"=w815:errorcluster)  [unwired: 7 in, 3 out]
        n328 = property class="niScope"(reference=w814, error in=w815, "Active Channel"=w813, "Channel Enabled"=FALSE ("Vertical:Channel Enabled")) -> (reference out=w804:refnum<k15>, error out=w805:errorcluster)
        n329 = call <instrlib>:"niScope Abort.vi"("instrument handle"=w804, "error in"=w805) -> ("error out"=w796:errorcluster)  [unwired: 12 in, 1 out]
        n330 = call "Pin Name to Reference.vim"("Pin Name"=w794, "type"=refnum<k15> refnum ("instrument handle"), "error in (no error)"=w796) -> ("Reference"=w799:refnum<k15>, "Channel"=w800:string, "error out"=w798:errorcluster)  [unwired: 7 in, 3 out]
        n331 = property class="niScope"(reference=w799, error in=w798, "Active Channel"=w800, "Channel Enabled"=FALSE ("Vertical:Channel Enabled")) -> (reference out=w803:refnum<k15>, error out=w802:errorcluster)
        n332 = call <instrlib>:"niScope Abort.vi"("instrument handle"=w803, "error in"=w802) -> ("error out"=w795:errorcluster)  [unwired: 12 in, 1 out]
      }
      frame "Test: Update UI" {
        # "If you want to update more indicators in the front panel do it here. It is efficient to update the UI in one case rather than in several cases. Also, it is a good practice to store the results in the data cluster in an efficient format and then get the data from data cluster and update the UI, in that way we could have the front panel independent of how we manipulate the data."
        n333 = call "Progress Monitor.vi"("State"=w825) -> ("State Array Index"=w827:i32)  [unwired: 14 in]
        n334 = property on="Progress" class="Slide (strict)"(error in=w826, "Value"=w827) -> (error out=w824:errorcluster)  [unwired: 1 in, 1 out]
        n335 = Unbundle By Name(w828) -> ("Test Results.Output Voltage Measured"=w818:T24, "Test Results.Input Voltage Measured"=w821:T24, "Test Results"=→"Test Results":T15, "Test Results.First Edge - Settling Time in s"=→"First Edge - Settling Time (s)":dbl, "Test Results.Second Edge - Settling Time in s"=→"Second Edge - Settling Time (s)":dbl)
        n336 = Build Array(w818, w821) -> (→"Line Transient":T5)
      }
      frame "Test: End" {
        # "End of the Test Procedure. Do cleanup of resources or references."
        n337 = call "Progress Monitor.vi"("State"=w830) -> ("State Array Index"=w833:i32)  [unwired: 14 in]
        n338 = property on="Progress" class="Slide (strict)"(error in=w831, "Value"=w833) -> (error out=w832:errorcluster)  [unwired: 1 in, 1 out]
      }
      frame "---------------------Misc-----------------------" {
      }
      frame "Error" {
        # "Handle the error and make sure to clear the error."
        n339 = Unbundle By Name(w842) -> ("Termination Monitor Info.Caller Information.Mode"=w841:T7)
        n340 = case shown="\"MeasurementSuite\"" w841 {
          tunnel: w845 -> [w849 w854 w856]
          tunnel: [w847 w851 w855] -> w843
          tunnel: [_ TRUE _] -> w840
          tunnel: w839 -> [_ w852 _]
          frame "Standalone" {
            w846 = T29 2 items=["no dialog", "OK message", "continue or stop message", "OK message + warnings", "continue/stop + warnings"] ("type of dialog (OK msg:1)")
            n341 = call <vilib>:"General Error Handler.vi"("type of dialog (OK msg:1)"=w846, "error in (no error)"=w849) -> ("error out"=w848:errorcluster)  [unwired: 9 in, 4 out]
            n342 = call <vilib>:"Clear Errors.vi"("error in (no error)"=w848) -> ("error out"=w847:errorcluster)  [unwired: 5 in, 1 out]
          }
          frame "Automation" {
            n343 = call <userlib>:"Release.vi"("Queue in"=w852) -> ("Error Out"=w850:errorcluster)  [unwired: 14 in]
            n344 = Merge Errors(w854, w850) -> (w851:errorcluster)
          }
          frame "MeasurementSuite" {
            n345 = property on="ErrorOccured" class="Clust (strict)"("Val(Sgnl)"=w856) -> (error out=w855:errorcluster)  [unwired: 2 in, 1 out]
          }
        }
      }
      frame "Exit" {
        # "Last case called before stopping the execution. \nError occured in this state will not be captured by Error state."
        n346 = call <userlib>:"Release.vi"("Queue in"=w862, "Error In"=w863) -> ("Error Out"=w858:errorcluster)  [unwired: 13 in]
        n347 = property on="Progress" class="Slide (strict)"(error in=w858, "Visible"=FALSE) -> (error out=w857:errorcluster)  [unwired: 1 in, 1 out]
      }
    }
  }
  "error out" <- w4
  "Header" <- "Line Transient" ("Header")
